vi "Autonomous Independent.vi"   [LabVIEW 2015]
doc: "This VI is called when autonomous begins, and will automatically be terminated when autonomous ends. You can carry out timed or sensor driven robot movement independently without needing to return to the caller."
uses:
  <vilib>/Rock Robotics/WPI/Solenoid/WPI_SolenoidValue.ctl
  <vilib>/Rock Robotics/WPI/Utilities/WPI_GetSetVariantRefNum.vi
  <vilib>/Rock Robotics/Network Tables/NT Read String.vi
  <vilib>/Rock Robotics/WPI/Solenoid/WPI_SolenoidSetEnum.vi
  Robot Global Data.vi
  <vilib>/Rock Robotics/Network Tables/NT Write Numeric Array.vi
panel:
  # "Be sure to right-click and choose Data Operations>>Make Current Value default if you want to save the array values with the VI"
types:
  T1 = typedef "WPI_JoystickDevRef.ctl" = cluster{"Device":T2}
  T2 = typedef "WPI_JoystickDeviceEnum.ctl" = enum16{"USB 0", "USB 1", "USB 2", "USB 3", "USB 4", "USB 5"}
  T3 = typedef "WPI_SolenoidValue.ctl" = enum16{"Off", "On", "Forward", "Reverse"}
  T4 = typedef "WPI_SolenoidDevRef.ctl" = cluster{"DevStatus":errorcluster, "Pneumatics Control Module":u8, "Forward Solenoid Channel":T5, "Reverse Solenoid Channel":T5}
  T5 = typedef "WPI_SolenoidChannel.ctl" = enum8{"Solenoid 0", "Solenoid 1", "Solenoid 2", "Solenoid 3", "Solenoid 4", "Solenoid 5", "Solenoid 6", "Solenoid 7", "Invalid"}
  T6 = typedef "WPI_RobotDriveDevRef.ctl" = cluster{"DevStatus":errorcluster, "Motors[]":T7[], "Square Inputs":bool, "Max Output":dbl}
  T7 = typedef "WPI_MotorControlDeviceRef.ctl" = cluster{"DeviceStatus":errorcluster, "Type":T8, "PWM":cluster{"PWM Channel":T9, "DeadBand":T10}, "CAN":cluster{"Device Number":u8, "Control Mode":T11, "Semaphore":T12, "Max Vout":dbl, "TalonSRX Control Mode":T13}, "Invert":bool}
  T8 = typedef "WPI_MotorControlType.ctl" = enum16{"PWM", "CAN", "CANTalonSRX"}
  T9 = typedef "FPGA_DIOPWMChannel.ctl" = enum8{"PWM 0", "PWM 1", "PWM 2", "PWM 3", "PWM 4", "PWM 5", "PWM 6", "PWM 7", "PWM 8", "PWM 9", "PWM MXP 0", "PWM MXP 1", "PWM MXP 2", "PWM MXP 3", "PWM MXP 4", "PWM MXP 5", "PWM MXP 6", "PWM MXP 7", "PWM MXP 8", "PWM MXP 9", "Invalid"}
  T10 = typedef "WPI_PWMDeadband.ctl" = cluster{"Name":string, "maxPositivePwm":i32, "minPositivePwm":i32, "centerPwm":i32, "maxNegativePwm":i32, "minNegativePwm":i32, "angularRange":u16}
  T11 = typedef "WPI_CANJaguar_ControlMode.ctl" = enum8{"Percent VBus", "Current", "Speed", "Position", "Voltage"}
  T12 = typedef "Semaphore RefNum" = refnum<k1>
  T13 = typedef "WPI_CANTalonSRX_APIControlMode.ctl" = enum8{"Percent VBus", "Speed", "Position", "Slave", "Unchanged / Invalid", "Voltage Compensation", "Current", "Motion Profile"}
  T14 = typedef "WPI_DigitalInputDevRef.ctl" = cluster{"DevStatus":errorcluster, "DIO Channel":T15}
  T15 = typedef "FPGA_DIOChannel.ctl" = enum8{"DIO 0", "DIO 1", "DIO 2", "DIO 3", "DIO 4", "DIO 5", "DIO 6", "DIO 7", "DIO 8", "DIO 9", "DIO MXP 0", "DIO MXP 1", "DIO MXP 2", "DIO MXP 3", "DIO MXP 4", "DIO MXP 5", "DIO MXP 6", "DIO MXP 7", "DIO MXP 8", "DIO MXP 9", "DIO MXP 10", "DIO MXP 11", "DIO MXP 12", "DIO MXP 13", "DIO MXP 14", "DIO MXP 15", "Invalid"}
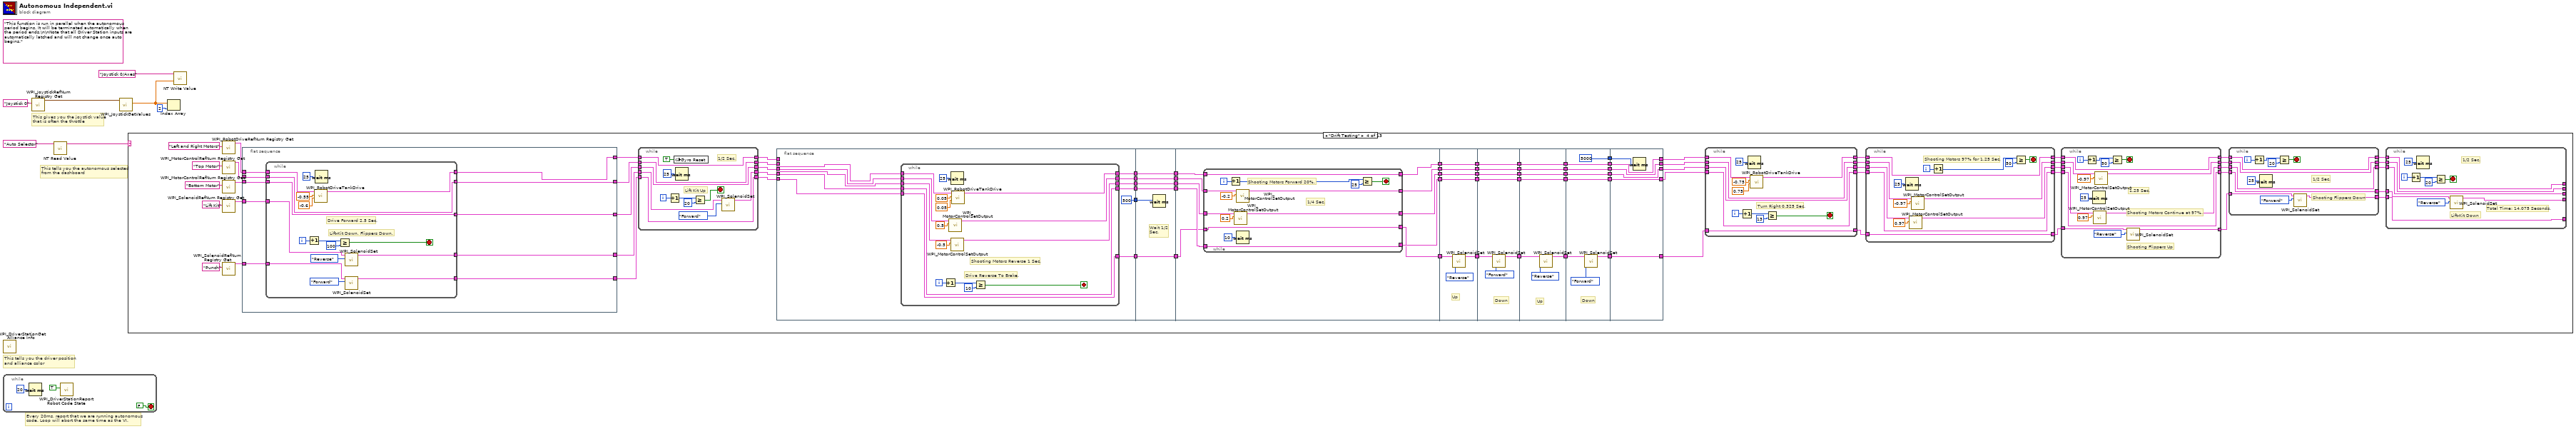
[diagram p0: block diagram]
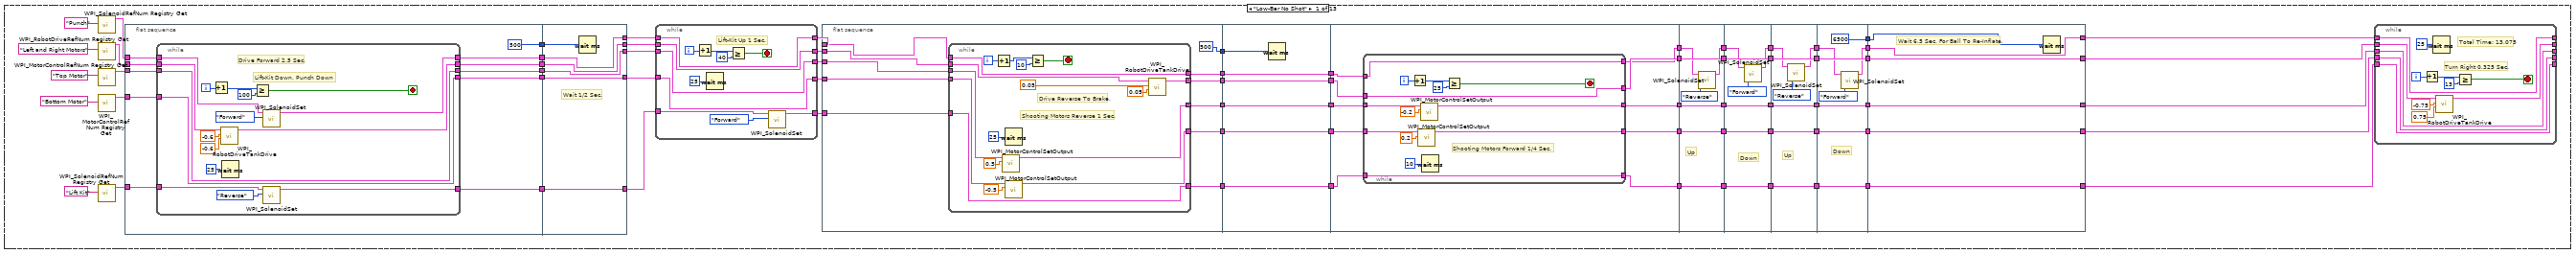
[diagram p2: hidden frame]
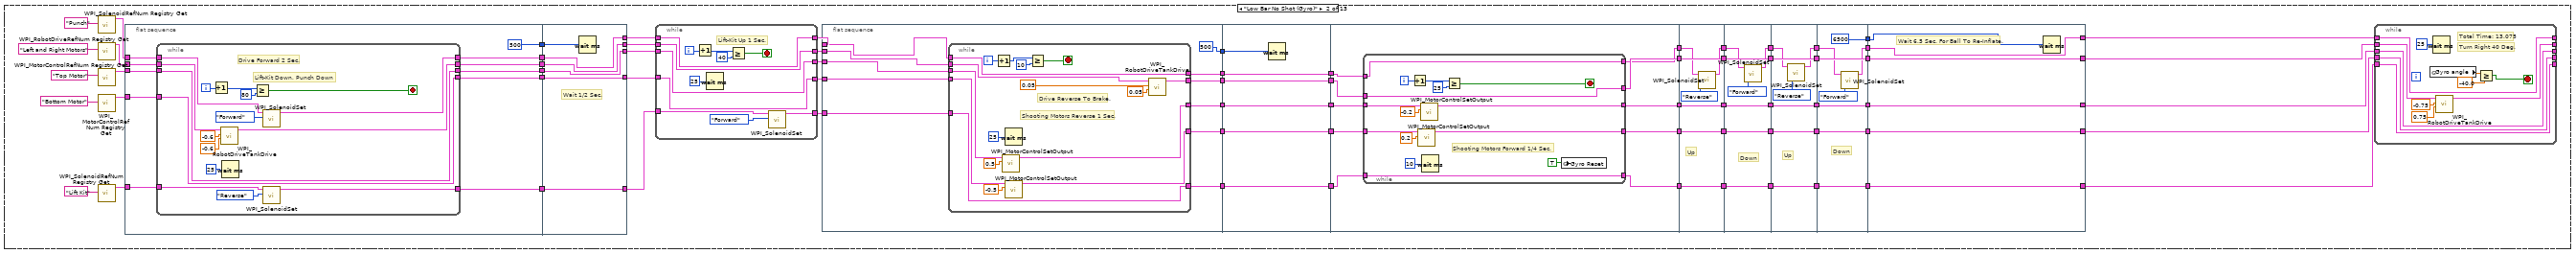
[diagram p3: hidden frame]
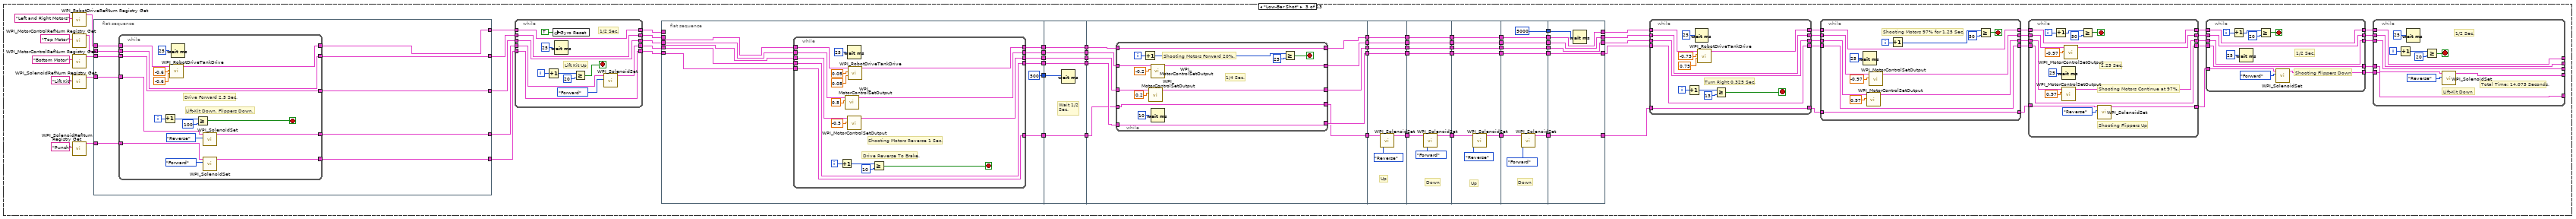
[diagram p4: hidden frame]
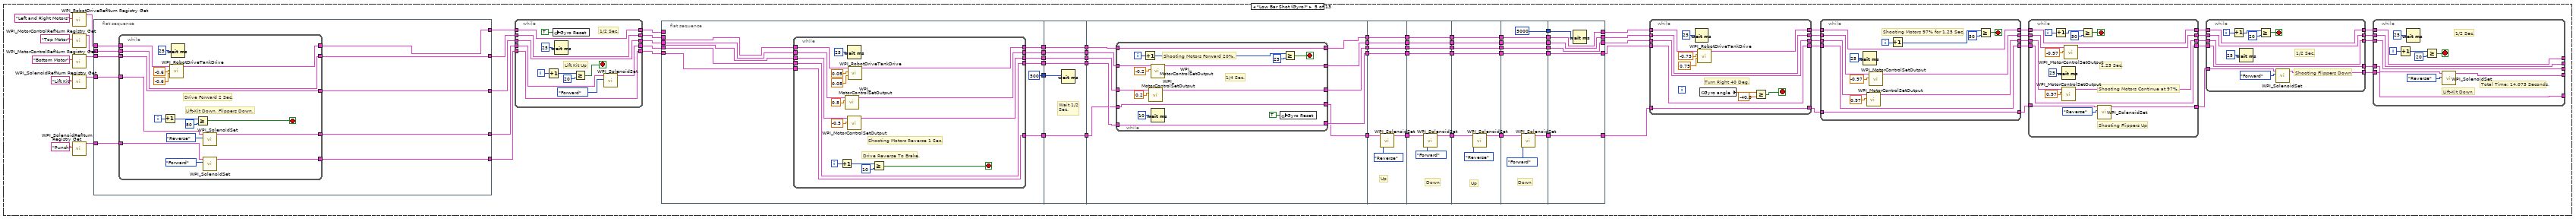
[diagram p5: hidden frame]
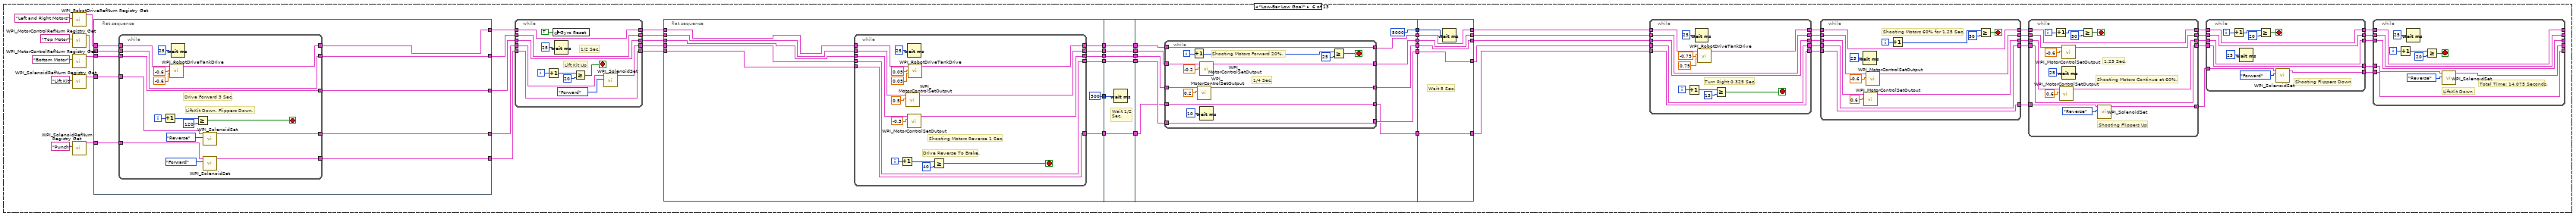
[diagram p6: hidden frame]
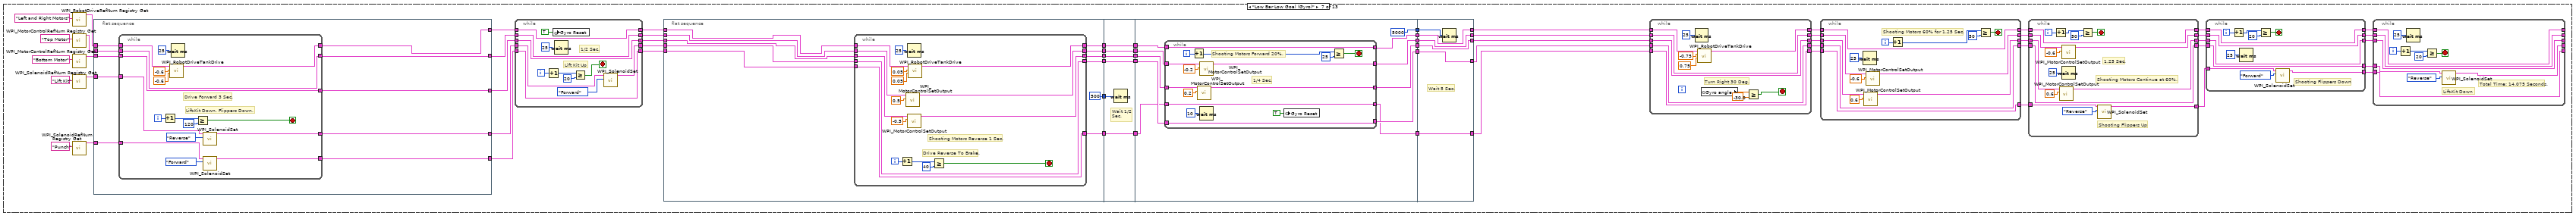
[diagram p7: hidden frame]
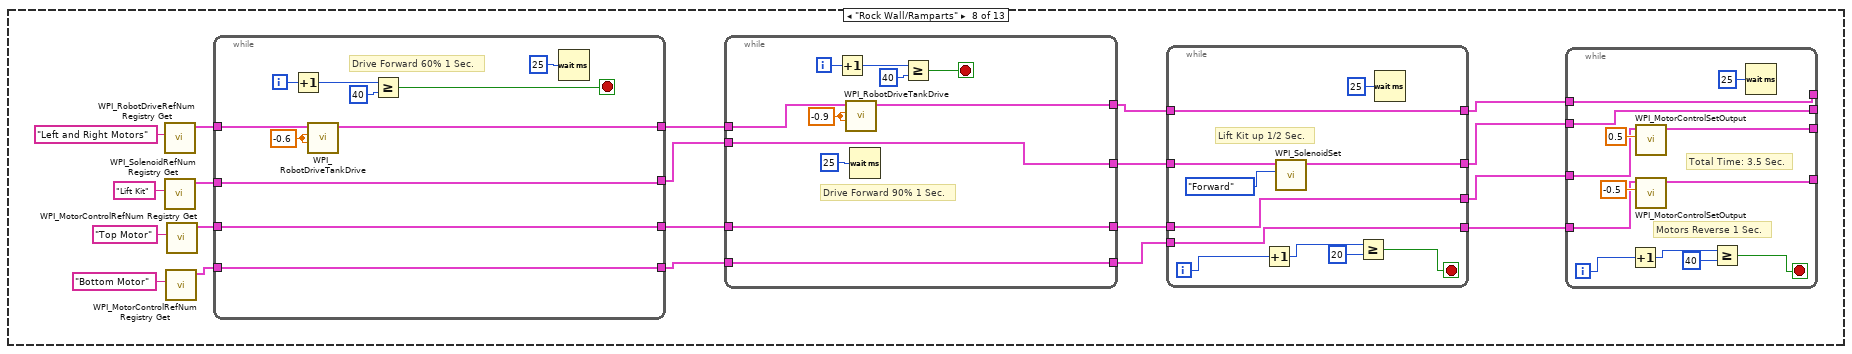
[diagram p8: hidden frame]
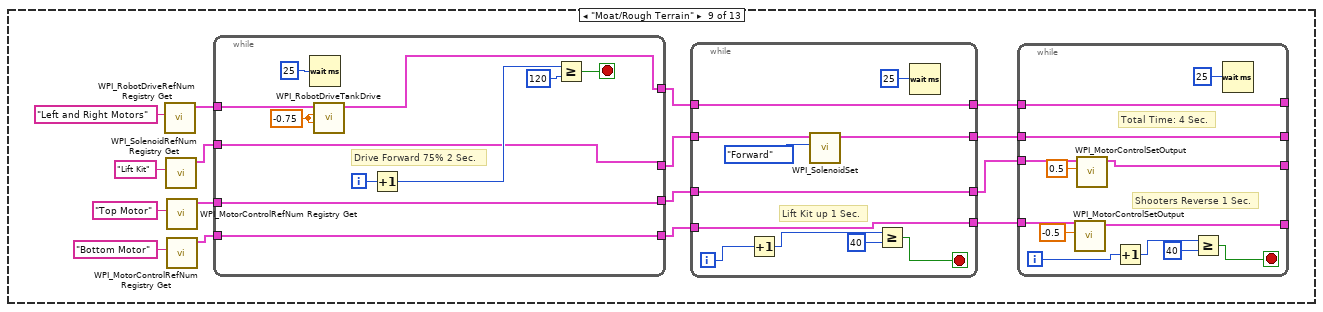
[diagram p9: hidden frame]
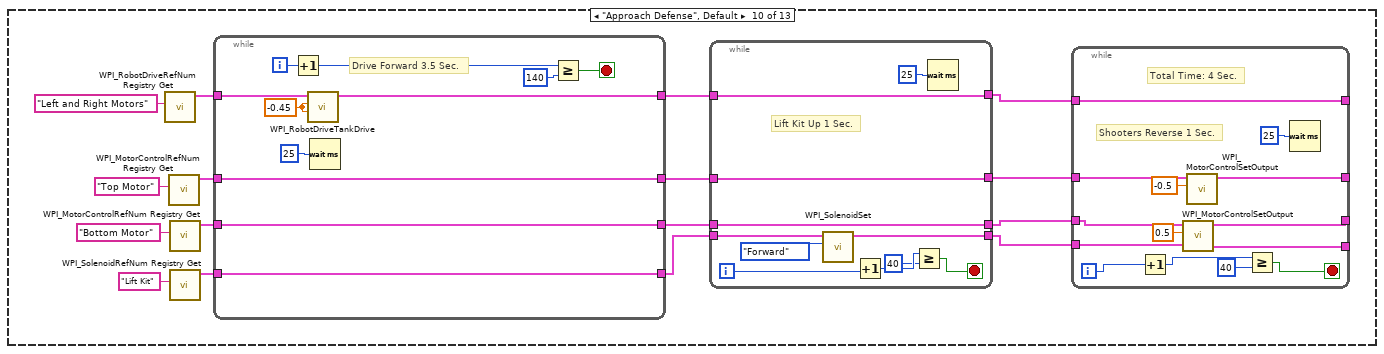
[diagram p10: hidden frame]
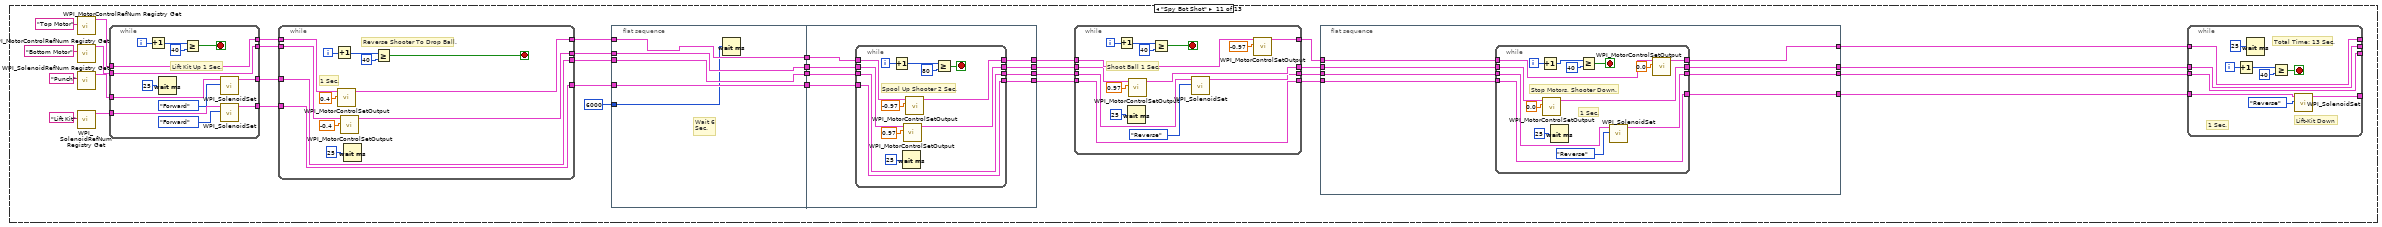
[diagram p11: hidden frame]
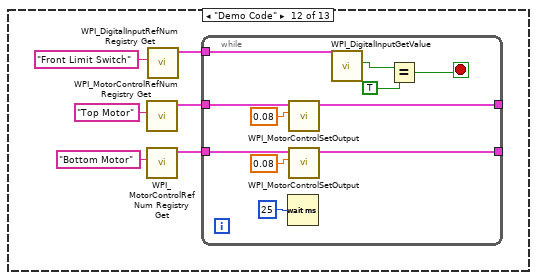
[diagram p12: hidden frame]
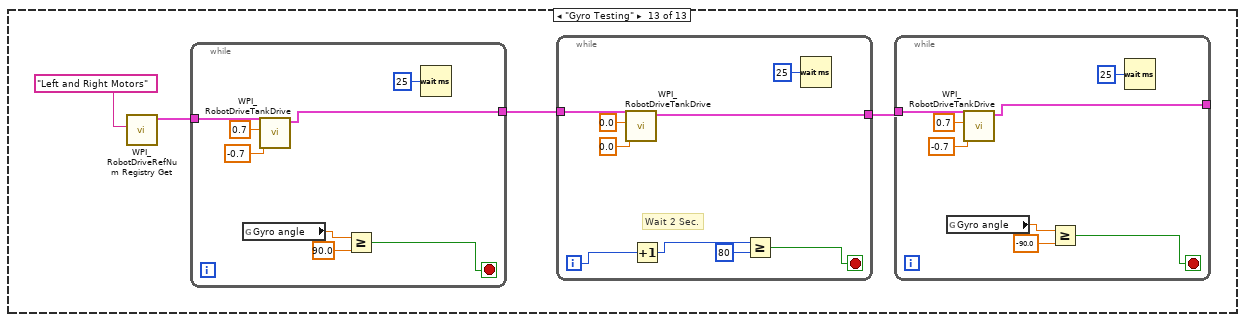
[diagram p13: hidden frame]
diagram:
  (unwired) "This function is run in parallel when the autonomous period begins. It will be terminated automatically when the period ends.\n\nNote that all Driver Station inputs are automatically latched and will not change once auto begins."
  # "This tells you the autonomous selected\nfrom the dashboard"
  # "Every 20ms, report that we are running autonomous\ncode. Loop will abort the same time as the VI."
  # "This gives you the joystick value\nthat is often the throttle"
  # "This tells you the driver position\nand alliance color"
  n1 = call <vilib>:"WPI_DriverStationGet Alliance Info.vi"() -> ()  [unwired: 12 out]
  n2 = while {
    stop <- FALSE stop-if-true
    n3 = Wait (ms)(milliseconds to wait=u32 20) -> ()  [unwired: 1 out]
    n4 = call <vilib>:"WPI_DriverStationReport Robot Code State.vi"("Autonomous"=TRUE) -> ()  [unwired: 10 in, 1 out]
  }
  n5 = call <vilib>:"WPI_JoystickRefNum Registry Get.vi"("refnum name"="Joystick 0") -> ("JoystickDevRef"=w6:T1)  [unwired: 1 in, 9 out]
  n6 = call-poly <vilib>:"NT Read Value.vi"("Name"="Auto Selector") -> ("String"=w3:string)  [unwired: 9 in, 1 out]
  n7 = call <vilib>:"WPI_JoystickGetValues.vi"("JoystickDevRef"=w6) -> ("Axes"=w2:dbl[])  [unwired: 6 in, 4 out]
  n8 = case shown="\"Drift Testing\"" w3 {
    frame "Low-Bar No Shot" {
      n9 = call <vilib>:"WPI_SolenoidRefNum Registry Get.vi"("refnum name"="Punch") -> ("SolenoidDevRef"=w70:T4)  [unwired: 9 in, 1 out]
      n10 = call <vilib>:"WPI_RobotDriveRefNum Registry Get.vi"("refnum name"="Left and Right Motors") -> ("RobotDriveDevRef"=w78:T6)  [unwired: 9 in, 1 out]
      n11 = call <vilib>:"WPI_MotorControlRefNum Registry Get.vi"("refnum name"="Top Motor") -> ("MotorControlDevRef"=w76:T7)  [unwired: 9 in, 1 out]
      n12 = call <vilib>:"WPI_MotorControlRefNum Registry Get.vi"("refnum name"="Bottom Motor") -> ("MotorControlDevRef"=w74:T7)  [unwired: 9 in, 1 out]
      n13 = call <vilib>:"WPI_SolenoidRefNum Registry Get.vi"("refnum name"="Lift Kit") -> ("SolenoidDevRef"=w72:T4)  [unwired: 9 in, 1 out]
      n14 = flat-sequence {
        tunnel: w78 -> [w89]
        tunnel: w76 -> [w87]
        tunnel: w74 -> [w85]
        tunnel: w72 -> [w83]
        tunnel: w70 -> [w81]
        tunnel: [w88] -> w53
        tunnel: [w86] -> w52
        tunnel: [w84] -> w51
        tunnel: [w82] -> w50
        tunnel: [w80] -> w49
        tunnel: [u32 500 ("milliseconds to wait")] -> w48
        tunnel: [w108] -> w69
        tunnel: [w109] -> w71
        tunnel: [w110] -> w73
        tunnel: [w111] -> w75
        tunnel: [w112] -> w77
        tunnel: w53 -> [w112]
        tunnel: w52 -> [w111]
        tunnel: w51 -> [w110]
        tunnel: w50 -> [w109]
        tunnel: w49 -> [w108]
        tunnel: w48 -> [w107]
        frame #0 {
          n15 = while {
            tunnel: w89 -> [w106]
            tunnel: [w99] -> w88
            tunnel: w87 -> [w97]
            tunnel: [w97] -> w86
            tunnel: w85 -> [w96]
            tunnel: [w96] -> w84
            tunnel: w83 -> [w95]
            tunnel: [w94] -> w82
            tunnel: [w90] -> w80
            tunnel: w81 -> [w91]
            i -> [w100]
            stop <- w101 stop-if-true
            # "Lift-Kit Down, Punch Down"
            # "Drive Forward 2.5 Sec."
            n16 = Increment(x=w100) -> (x+1=w103:i32)
            n17 = call <vilib>:"WPI_RobotDriveTankDrive.vi"("Right axis value"=-0.6, "Left axis value"=-0.6, "RobotDriveDevRef"=w106) -> ("RobotDriveDevRef"=w99:T6)  [unwired: 6 in, 2 out]
            n18 = Wait (ms)(milliseconds to wait=u32 25) -> ()  [unwired: 1 out]
            n19 = Greater Or Equal?(x=w103, y=100) -> (x >= y?=w101:bool)
            n20 = call-poly <vilib>:"WPI_SolenoidSet.vi"("Value"=WPI_SolenoidValue."Forward", "SolenoidDevRef"=w91) -> ("SolenoidDevRef"=w90:T4)  [unwired: 8 in, 1 out]
            n21 = call-poly <vilib>:"WPI_SolenoidSet.vi"("Value"=WPI_SolenoidValue."Reverse", "SolenoidDevRef"=w95) -> ("SolenoidDevRef"=w94:T4)  [unwired: 8 in, 1 out]
          }
        }
        frame #1 {
          # "Wait 1/2 Sec."
          n22 = Wait (ms)(milliseconds to wait=w107) -> ()  [unwired: 1 out]
        }
      }
      n23 = while {
        tunnel: [w217] -> w68
        tunnel: w77 -> [w217]
        tunnel: [w211] -> w64
        tunnel: w75 -> [w211]
        tunnel: [w210] -> w63
        tunnel: w73 -> [w210]
        tunnel: w71 -> [w208]
        tunnel: [w207] -> w62
        tunnel: w69 -> [w206]
        tunnel: [w206] -> w66
        i -> [w213]
        stop <- w214 stop-if-true
        # "Lift-Kit Up 1 Sec."
        n24 = Increment(x=w213) -> (x+1=w215:i32)
        n25 = Wait (ms)(milliseconds to wait=u32 25) -> ()  [unwired: 1 out]
        n26 = Greater Or Equal?(x=w215, y=40) -> (x >= y?=w214:bool)
        n27 = call-poly <vilib>:"WPI_SolenoidSet.vi"("Value"=WPI_SolenoidValue."Forward", "SolenoidDevRef"=w208) -> ("SolenoidDevRef"=w207:T4)  [unwired: 8 in, 1 out]
      }
      n28 = flat-sequence {
        tunnel: [w122] -> w47
        tunnel: [w121] -> w45
        tunnel: [w117] -> w43
        tunnel: [w116] -> w41
        tunnel: [w115] -> w39
        tunnel: [u32 500 ("milliseconds to wait")] -> w37
        tunnel: w62 -> [w118]
        tunnel: w63 -> [w119]
        tunnel: w64 -> [w120]
        tunnel: w66 -> [w114]
        tunnel: w68 -> [w123]
        tunnel: w47 -> [w146]
        tunnel: [w146] -> w46
        tunnel: w45 -> [w145]
        tunnel: [w145] -> w44
        tunnel: w43 -> [w144]
        tunnel: [w144] -> w42
        tunnel: w41 -> [w143]
        tunnel: [w143] -> w40
        tunnel: w39 -> [w142]
        tunnel: [w142] -> w38
        tunnel: w37 -> [w141]
        tunnel: w46 -> [w152]
        tunnel: [w151] -> w36
        tunnel: w44 -> [w150]
        tunnel: [w149] -> w35
        tunnel: w42 -> [w148]
        tunnel: [w147] -> w34
        tunnel: w40 -> [w156]
        tunnel: [w154] -> w33
        tunnel: w38 -> [w155]
        tunnel: [w153] -> w32
        tunnel: w36 -> [w177]
        tunnel: [w177] -> w31
        tunnel: w35 -> [w176]
        tunnel: [w172] -> w30
        tunnel: w34 -> [w175]
        tunnel: [w175] -> w29
        tunnel: w33 -> [w174]
        tunnel: [w174] -> w28
        tunnel: w32 -> [w173]
        tunnel: [w173] -> w27
        tunnel: w31 -> [w184]
        tunnel: [w184] -> w26
        tunnel: w30 -> [w183]
        tunnel: [w179] -> w25
        tunnel: w29 -> [w182]
        tunnel: [w182] -> w24
        tunnel: w28 -> [w181]
        tunnel: [w181] -> w23
        tunnel: w27 -> [w180]
        tunnel: [w180] -> w22
        tunnel: w26 -> [w191]
        tunnel: [w191] -> w21
        tunnel: w25 -> [w190]
        tunnel: [w186] -> w19
        tunnel: w24 -> [w189]
        tunnel: [w189] -> w17
        tunnel: w23 -> [w188]
        tunnel: [w188] -> w15
        tunnel: w22 -> [w187]
        tunnel: [w187] -> w13
        tunnel: w21 -> [w199]
        tunnel: [w199] -> w20
        tunnel: w19 -> [w198]
        tunnel: [w194] -> w18
        tunnel: w17 -> [w197]
        tunnel: [w197] -> w16
        tunnel: w15 -> [w196]
        tunnel: [w196] -> w14
        tunnel: w13 -> [w195]
        tunnel: [w195] -> w12
        tunnel: [u32 6500 ("milliseconds to wait")] -> w11
        tunnel: [w201] -> w59
        tunnel: [w202] -> w60
        tunnel: [w203] -> w61
        tunnel: [w204] -> w65
        tunnel: [w205] -> w67
        tunnel: w20 -> [w205]
        tunnel: w18 -> [w204]
        tunnel: w16 -> [w203]
        tunnel: w14 -> [w202]
        tunnel: w12 -> [w201]
        tunnel: w11 -> [w200]
        frame #0 {
          n29 = while {
            tunnel: [w127] -> w122
            tunnel: w123 -> [w140]
            tunnel: [w124] -> w121
            tunnel: w114 -> [w124]
            tunnel: w120 -> [w139]
            tunnel: w119 -> [w138]
            tunnel: [w135] -> w117
            tunnel: w118 -> [w135]
            tunnel: [w134] -> w116
            tunnel: [w133] -> w115
            i -> [w129]
            stop <- w128 stop-if-true
            # "Drive Reverse To Brake."
            # "Shooting Motors Reverse 1 Sec."
            n30 = Increment(x=w129) -> (x+1=w131:i32)
            n31 = call <vilib>:"WPI_MotorControlSetOutput.vi"("Output"=0.5, "MotorControlDevRef"=w139) -> ("MotorControlDevRef"=w134:T7)  [unwired: 7 in, 2 out]
            n32 = Wait (ms)(milliseconds to wait=u32 25) -> ()  [unwired: 1 out]
            n33 = call <vilib>:"WPI_MotorControlSetOutput.vi"("Output"=-0.5, "MotorControlDevRef"=w138) -> ("MotorControlDevRef"=w133:T7)  [unwired: 7 in, 2 out]
            n34 = Greater Or Equal?(x=w131, y=10) -> (x >= y?=w128:bool)
            n35 = call <vilib>:"WPI_RobotDriveTankDrive.vi"("Right axis value"=0.05, "Left axis value"=0.05, "RobotDriveDevRef"=w140) -> ("RobotDriveDevRef"=w127:T6)  [unwired: 6 in, 2 out]
          }
        }
        frame #1 {
          n36 = Wait (ms)(milliseconds to wait=w141) -> ()  [unwired: 1 out]
        }
        frame #2 {
          n37 = while {
            tunnel: w156 -> [w170]
            tunnel: w155 -> [w169]
            tunnel: [w161] -> w154
            tunnel: [w160] -> w153
            tunnel: [w159] -> w151
            tunnel: w152 -> [w159]
            tunnel: [w158] -> w149
            tunnel: w150 -> [w158]
            tunnel: [w157] -> w147
            tunnel: w148 -> [w157]
            i -> [w165]
            stop <- w162 stop-if-true
            # "Shooting Motors Forward 1/4 Sec."
            n38 = Increment(x=w165) -> (x+1=w164:i32)
            n39 = call <vilib>:"WPI_MotorControlSetOutput.vi"("Output"=0.2, "MotorControlDevRef"=w169) -> ("MotorControlDevRef"=w160:T7)  [unwired: 7 in, 2 out]
            n40 = call <vilib>:"WPI_MotorControlSetOutput.vi"("Output"=-0.2, "MotorControlDevRef"=w170) -> ("MotorControlDevRef"=w161:T7)  [unwired: 7 in, 2 out]
            n41 = Wait (ms)(milliseconds to wait=u32 10) -> ()  [unwired: 1 out]
            n42 = Greater Or Equal?(x=w164, y=25) -> (x >= y?=w162:bool)
          }
        }
        frame #3 {
          # "Up"
          n43 = call-poly <vilib>:"WPI_SolenoidSet.vi"("Value"=WPI_SolenoidValue."Reverse", "SolenoidDevRef"=w176) -> ("SolenoidDevRef"=w172:T4)  [unwired: 8 in, 1 out]
        }
        frame #4 {
          # "Down"
          n44 = call-poly <vilib>:"WPI_SolenoidSet.vi"("Value"=WPI_SolenoidValue."Forward", "SolenoidDevRef"=w183) -> ("SolenoidDevRef"=w179:T4)  [unwired: 8 in, 1 out]
        }
        frame #5 {
          # "Up"
          n45 = call-poly <vilib>:"WPI_SolenoidSet.vi"("Value"=WPI_SolenoidValue."Reverse", "SolenoidDevRef"=w190) -> ("SolenoidDevRef"=w186:T4)  [unwired: 8 in, 1 out]
        }
        frame #6 {
          # "Down"
          n46 = call-poly <vilib>:"WPI_SolenoidSet.vi"("Value"=WPI_SolenoidValue."Forward", "SolenoidDevRef"=w198) -> ("SolenoidDevRef"=w194:T4)  [unwired: 8 in, 1 out]
        }
        frame #7 {
          # "Wait 6.5 Sec. For Ball To Re-Inflate."
          n47 = Wait (ms)(milliseconds to wait=w200) -> ()  [unwired: 1 out]
        }
      }
      n48 = while {
        tunnel: w67 -> [w230]
        tunnel: w60 -> [w226]
        tunnel: [w226] -> _
        tunnel: [w225] -> _
        tunnel: w59 -> [w225]
        tunnel: [w224] -> _
        tunnel: [w223] -> _
        tunnel: w61 -> [w223]
        tunnel: [w222] -> _
        tunnel: w65 -> [w222]
        i -> [w220]
        stop <- w218 stop-if-true
        # "Total Time: 13.075"
        # "Turn Right 0.325 Sec."
        n49 = Increment(x=w220) -> (x+1=w221:i32)
        n50 = Wait (ms)(milliseconds to wait=u32 25) -> ()  [unwired: 1 out]
        n51 = call <vilib>:"WPI_RobotDriveTankDrive.vi"("Right axis value"=0.75, "Left axis value"=-0.75, "RobotDriveDevRef"=w230) -> ("RobotDriveDevRef"=w224:T6)  [unwired: 6 in, 2 out]
        n52 = Greater Or Equal?(x=w221, y=13) -> (x >= y?=w218:bool)
      }
    }
    frame "Low Bar No Shot (Gyro)" {
      n53 = call <vilib>:"WPI_SolenoidRefNum Registry Get.vi"("refnum name"="Punch") -> ("SolenoidDevRef"=w290:T4)  [unwired: 9 in, 1 out]
      n54 = call <vilib>:"WPI_RobotDriveRefNum Registry Get.vi"("refnum name"="Left and Right Motors") -> ("RobotDriveDevRef"=w298:T6)  [unwired: 9 in, 1 out]
      n55 = call <vilib>:"WPI_MotorControlRefNum Registry Get.vi"("refnum name"="Top Motor") -> ("MotorControlDevRef"=w296:T7)  [unwired: 9 in, 1 out]
      n56 = call <vilib>:"WPI_MotorControlRefNum Registry Get.vi"("refnum name"="Bottom Motor") -> ("MotorControlDevRef"=w294:T7)  [unwired: 9 in, 1 out]
      n57 = call <vilib>:"WPI_SolenoidRefNum Registry Get.vi"("refnum name"="Lift Kit") -> ("SolenoidDevRef"=w292:T4)  [unwired: 9 in, 1 out]
      n58 = flat-sequence {
        tunnel: w298 -> [w309]
        tunnel: w296 -> [w307]
        tunnel: w294 -> [w305]
        tunnel: w292 -> [w303]
        tunnel: w290 -> [w301]
        tunnel: [w308] -> w273
        tunnel: [w306] -> w272
        tunnel: [w304] -> w271
        tunnel: [w302] -> w270
        tunnel: [w300] -> w269
        tunnel: [u32 500 ("milliseconds to wait")] -> w268
        tunnel: [w328] -> w289
        tunnel: [w329] -> w291
        tunnel: [w330] -> w293
        tunnel: [w331] -> w295
        tunnel: [w332] -> w297
        tunnel: w273 -> [w332]
        tunnel: w272 -> [w331]
        tunnel: w271 -> [w330]
        tunnel: w270 -> [w329]
        tunnel: w269 -> [w328]
        tunnel: w268 -> [w327]
        frame #0 {
          n59 = while {
            tunnel: w309 -> [w326]
            tunnel: [w319] -> w308
            tunnel: w307 -> [w317]
            tunnel: [w317] -> w306
            tunnel: w305 -> [w316]
            tunnel: [w316] -> w304
            tunnel: w303 -> [w315]
            tunnel: [w314] -> w302
            tunnel: [w310] -> w300
            tunnel: w301 -> [w311]
            i -> [w320]
            stop <- w321 stop-if-true
            # "Lift-Kit Down, Punch Down"
            # "Drive Forward 2 Sec."
            n60 = Increment(x=w320) -> (x+1=w323:i32)
            n61 = call <vilib>:"WPI_RobotDriveTankDrive.vi"("Right axis value"=-0.6, "Left axis value"=-0.6, "RobotDriveDevRef"=w326) -> ("RobotDriveDevRef"=w319:T6)  [unwired: 6 in, 2 out]
            n62 = Wait (ms)(milliseconds to wait=u32 25) -> ()  [unwired: 1 out]
            n63 = Greater Or Equal?(x=w323, y=80) -> (x >= y?=w321:bool)
            n64 = call-poly <vilib>:"WPI_SolenoidSet.vi"("Value"=WPI_SolenoidValue."Forward", "SolenoidDevRef"=w311) -> ("SolenoidDevRef"=w310:T4)  [unwired: 8 in, 1 out]
            n65 = call-poly <vilib>:"WPI_SolenoidSet.vi"("Value"=WPI_SolenoidValue."Reverse", "SolenoidDevRef"=w315) -> ("SolenoidDevRef"=w314:T4)  [unwired: 8 in, 1 out]
          }
        }
        frame #1 {
          # "Wait 1/2 Sec."
          n66 = Wait (ms)(milliseconds to wait=w327) -> ()  [unwired: 1 out]
        }
      }
      n67 = while {
        tunnel: [w438] -> w288
        tunnel: w297 -> [w438]
        tunnel: [w432] -> w284
        tunnel: w295 -> [w432]
        tunnel: [w431] -> w283
        tunnel: w293 -> [w431]
        tunnel: w291 -> [w429]
        tunnel: [w428] -> w282
        tunnel: w289 -> [w427]
        tunnel: [w427] -> w286
        i -> [w434]
        stop <- w435 stop-if-true
        # "Lift-Kit Up 1 Sec."
        n68 = Increment(x=w434) -> (x+1=w436:i32)
        n69 = Wait (ms)(milliseconds to wait=u32 25) -> ()  [unwired: 1 out]
        n70 = Greater Or Equal?(x=w436, y=40) -> (x >= y?=w435:bool)
        n71 = call-poly <vilib>:"WPI_SolenoidSet.vi"("Value"=WPI_SolenoidValue."Forward", "SolenoidDevRef"=w429) -> ("SolenoidDevRef"=w428:T4)  [unwired: 8 in, 1 out]
      }
      n72 = flat-sequence {
        tunnel: [w342] -> w267
        tunnel: [w341] -> w265
        tunnel: [w337] -> w263
        tunnel: [w336] -> w261
        tunnel: [w335] -> w259
        tunnel: [u32 500 ("milliseconds to wait")] -> w257
        tunnel: w282 -> [w338]
        tunnel: w283 -> [w339]
        tunnel: w284 -> [w340]
        tunnel: w286 -> [w334]
        tunnel: w288 -> [w343]
        tunnel: w267 -> [w366]
        tunnel: [w366] -> w266
        tunnel: w265 -> [w365]
        tunnel: [w365] -> w264
        tunnel: w263 -> [w364]
        tunnel: [w364] -> w262
        tunnel: w261 -> [w363]
        tunnel: [w363] -> w260
        tunnel: w259 -> [w362]
        tunnel: [w362] -> w258
        tunnel: w257 -> [w361]
        tunnel: w266 -> [w372]
        tunnel: [w371] -> w256
        tunnel: w264 -> [w370]
        tunnel: [w369] -> w255
        tunnel: w262 -> [w368]
        tunnel: [w367] -> w254
        tunnel: w260 -> [w376]
        tunnel: [w374] -> w253
        tunnel: w258 -> [w375]
        tunnel: [w373] -> w252
        tunnel: w256 -> [w398]
        tunnel: [w398] -> w251
        tunnel: w255 -> [w397]
        tunnel: [w393] -> w250
        tunnel: w254 -> [w396]
        tunnel: [w396] -> w249
        tunnel: w253 -> [w395]
        tunnel: [w395] -> w248
        tunnel: w252 -> [w394]
        tunnel: [w394] -> w247
        tunnel: w251 -> [w405]
        tunnel: [w405] -> w246
        tunnel: w250 -> [w404]
        tunnel: [w400] -> w245
        tunnel: w249 -> [w403]
        tunnel: [w403] -> w244
        tunnel: w248 -> [w402]
        tunnel: [w402] -> w243
        tunnel: w247 -> [w401]
        tunnel: [w401] -> w242
        tunnel: w246 -> [w412]
        tunnel: [w412] -> w241
        tunnel: w245 -> [w411]
        tunnel: [w407] -> w239
        tunnel: w244 -> [w410]
        tunnel: [w410] -> w237
        tunnel: w243 -> [w409]
        tunnel: [w409] -> w235
        tunnel: w242 -> [w408]
        tunnel: [w408] -> w233
        tunnel: w241 -> [w420]
        tunnel: [w420] -> w240
        tunnel: w239 -> [w419]
        tunnel: [w415] -> w238
        tunnel: w237 -> [w418]
        tunnel: [w418] -> w236
        tunnel: w235 -> [w417]
        tunnel: [w417] -> w234
        tunnel: w233 -> [w416]
        tunnel: [w416] -> w232
        tunnel: [u32 6500 ("milliseconds to wait")] -> w231
        tunnel: [w422] -> w279
        tunnel: [w423] -> w280
        tunnel: [w424] -> w281
        tunnel: [w425] -> w285
        tunnel: [w426] -> w287
        tunnel: w240 -> [w426]
        tunnel: w238 -> [w425]
        tunnel: w236 -> [w424]
        tunnel: w234 -> [w423]
        tunnel: w232 -> [w422]
        tunnel: w231 -> [w421]
        frame #0 {
          n73 = while {
            tunnel: [w347] -> w342
            tunnel: w343 -> [w360]
            tunnel: [w344] -> w341
            tunnel: w334 -> [w344]
            tunnel: w340 -> [w359]
            tunnel: w339 -> [w358]
            tunnel: [w355] -> w337
            tunnel: w338 -> [w355]
            tunnel: [w354] -> w336
            tunnel: [w353] -> w335
            i -> [w349]
            stop <- w348 stop-if-true
            # "Drive Reverse To Brake."
            # "Shooting Motors Reverse 1 Sec."
            n74 = Increment(x=w349) -> (x+1=w351:i32)
            n75 = call <vilib>:"WPI_MotorControlSetOutput.vi"("Output"=0.5, "MotorControlDevRef"=w359) -> ("MotorControlDevRef"=w354:T7)  [unwired: 7 in, 2 out]
            n76 = Wait (ms)(milliseconds to wait=u32 25) -> ()  [unwired: 1 out]
            n77 = call <vilib>:"WPI_MotorControlSetOutput.vi"("Output"=-0.5, "MotorControlDevRef"=w358) -> ("MotorControlDevRef"=w353:T7)  [unwired: 7 in, 2 out]
            n78 = Greater Or Equal?(x=w351, y=10) -> (x >= y?=w348:bool)
            n79 = call <vilib>:"WPI_RobotDriveTankDrive.vi"("Right axis value"=0.05, "Left axis value"=0.05, "RobotDriveDevRef"=w360) -> ("RobotDriveDevRef"=w347:T6)  [unwired: 6 in, 2 out]
          }
        }
        frame #1 {
          n80 = Wait (ms)(milliseconds to wait=w361) -> ()  [unwired: 1 out]
        }
        frame #2 {
          n81 = while {
            tunnel: w376 -> [w391]
            tunnel: w375 -> [w390]
            tunnel: [w382] -> w374
            tunnel: [w381] -> w373
            tunnel: [w380] -> w371
            tunnel: w372 -> [w380]
            tunnel: [w379] -> w369
            tunnel: w370 -> [w379]
            tunnel: [w378] -> w367
            tunnel: w368 -> [w378]
            i -> [w386]
            stop <- w383 stop-if-true
            # "Shooting Motors Forward 1/4 Sec."
            n82 = Increment(x=w386) -> (x+1=w385:i32)
            n83 = call <vilib>:"WPI_MotorControlSetOutput.vi"("Output"=0.2, "MotorControlDevRef"=w390) -> ("MotorControlDevRef"=w381:T7)  [unwired: 7 in, 2 out]
            n84 = call <vilib>:"WPI_MotorControlSetOutput.vi"("Output"=-0.2, "MotorControlDevRef"=w391) -> ("MotorControlDevRef"=w382:T7)  [unwired: 7 in, 2 out]
            n85 = Wait (ms)(milliseconds to wait=u32 10) -> ()  [unwired: 1 out]
            n86 = Greater Or Equal?(x=w385, y=25) -> (x >= y?=w383:bool)
            n87 = global write "Robot Global Data.vi" "Gyro Reset"(TRUE ("Gyro Reset")) -> ()
          }
        }
        frame #3 {
          # "Up"
          n88 = call-poly <vilib>:"WPI_SolenoidSet.vi"("Value"=WPI_SolenoidValue."Reverse", "SolenoidDevRef"=w397) -> ("SolenoidDevRef"=w393:T4)  [unwired: 8 in, 1 out]
        }
        frame #4 {
          # "Down"
          n89 = call-poly <vilib>:"WPI_SolenoidSet.vi"("Value"=WPI_SolenoidValue."Forward", "SolenoidDevRef"=w404) -> ("SolenoidDevRef"=w400:T4)  [unwired: 8 in, 1 out]
        }
        frame #5 {
          # "Up"
          n90 = call-poly <vilib>:"WPI_SolenoidSet.vi"("Value"=WPI_SolenoidValue."Reverse", "SolenoidDevRef"=w411) -> ("SolenoidDevRef"=w407:T4)  [unwired: 8 in, 1 out]
        }
        frame #6 {
          # "Down"
          n91 = call-poly <vilib>:"WPI_SolenoidSet.vi"("Value"=WPI_SolenoidValue."Forward", "SolenoidDevRef"=w419) -> ("SolenoidDevRef"=w415:T4)  [unwired: 8 in, 1 out]
        }
        frame #7 {
          # "Wait 6.5 Sec. For Ball To Re-Inflate."
          n92 = Wait (ms)(milliseconds to wait=w421) -> ()  [unwired: 1 out]
        }
      }
      n93 = while {
        tunnel: w287 -> [w450]
        tunnel: w280 -> [w446]
        tunnel: [w446] -> _
        tunnel: [w445] -> _
        tunnel: w279 -> [w445]
        tunnel: [w444] -> _
        tunnel: [w443] -> _
        tunnel: w281 -> [w443]
        tunnel: [w442] -> _
        tunnel: w285 -> [w442]
        stop <- w440 stop-if-true
        # "Total Time: 13.075"
        # "Turn Right 40 Deg."
        n94 = global read "Robot Global Data.vi" "Gyro angle"() -> (w441:dbl)
        n95 = Wait (ms)(milliseconds to wait=u32 25) -> ()  [unwired: 1 out]
        n96 = call <vilib>:"WPI_RobotDriveTankDrive.vi"("Right axis value"=0.75, "Left axis value"=-0.75, "RobotDriveDevRef"=w450) -> ("RobotDriveDevRef"=w444:T6)  [unwired: 6 in, 2 out]
        n97 = Greater Or Equal?(x=w441, y=-40.0) -> (x >= y?=w440:bool)
      }
    }
    frame "Low-Bar Shot" {
      n98 = call <vilib>:"WPI_RobotDriveRefNum Registry Get.vi"("refnum name"="Left and Right Motors") -> ("RobotDriveDevRef"=w532:T6)  [unwired: 9 in, 1 out]
      n99 = call <vilib>:"WPI_MotorControlRefNum Registry Get.vi"("refnum name"="Top Motor") -> ("MotorControlDevRef"=w528:T7)  [unwired: 9 in, 1 out]
      n100 = call <vilib>:"WPI_MotorControlRefNum Registry Get.vi"("refnum name"="Bottom Motor") -> ("MotorControlDevRef"=w526:T7)  [unwired: 9 in, 1 out]
      n101 = call <vilib>:"WPI_SolenoidRefNum Registry Get.vi"("refnum name"="Lift Kit") -> ("SolenoidDevRef"=w523:T4)  [unwired: 9 in, 1 out]
      n102 = call <vilib>:"WPI_SolenoidRefNum Registry Get.vi"("refnum name"="Punch") -> ("SolenoidDevRef"=w520:T4)  [unwired: 9 in, 1 out]
      n103 = flat-sequence {
        tunnel: [w550] -> w519
        tunnel: [w551] -> w522
        tunnel: [w552] -> w525
        tunnel: [w553] -> w527
        tunnel: [w554] -> w529
        tunnel: w520 -> [w545]
        tunnel: w523 -> [w546]
        tunnel: w526 -> [w547]
        tunnel: w528 -> [w548]
        tunnel: w532 -> [w549]
        frame #0 {
          n104 = while {
            tunnel: w549 -> [w571]
            tunnel: [w564] -> w554
            tunnel: w548 -> [w562]
            tunnel: [w562] -> w553
            tunnel: w547 -> [w561]
            tunnel: [w561] -> w552
            tunnel: w546 -> [w560]
            tunnel: [w559] -> w551
            tunnel: [w555] -> w550
            tunnel: w545 -> [w556]
            i -> [w565]
            stop <- w566 stop-if-true
            # "Lift-Kit Down, Flippers Down."
            # "Drive Forward 2.5 Sec."
            n105 = Increment(x=w565) -> (x+1=w568:i32)
            n106 = call <vilib>:"WPI_RobotDriveTankDrive.vi"("Right axis value"=-0.6, "Left axis value"=-0.6, "RobotDriveDevRef"=w571) -> ("RobotDriveDevRef"=w564:T6)  [unwired: 6 in, 2 out]
            n107 = Wait (ms)(milliseconds to wait=u32 25) -> ()  [unwired: 1 out]
            n108 = Greater Or Equal?(x=w568, y=100) -> (x >= y?=w566:bool)
            n109 = call-poly <vilib>:"WPI_SolenoidSet.vi"("Value"=WPI_SolenoidValue."Reverse", "SolenoidDevRef"=w560) -> ("SolenoidDevRef"=w559:T4)  [unwired: 8 in, 1 out]
            n110 = call-poly <vilib>:"WPI_SolenoidSet.vi"("Value"=WPI_SolenoidValue."Forward", "SolenoidDevRef"=w556) -> ("SolenoidDevRef"=w555:T4)  [unwired: 8 in, 1 out]
          }
        }
      }
      n111 = while {
        tunnel: [w689] -> w509
        tunnel: w529 -> [w689]
        tunnel: [w682] -> w506
        tunnel: w527 -> [w682]
        tunnel: [w681] -> w505
        tunnel: w525 -> [w681]
        tunnel: w522 -> [w679]
        tunnel: [w678] -> w504
        tunnel: w519 -> [w677]
        tunnel: [w677] -> w507
        i -> [w684]
        stop <- w685 stop-if-true
        # "1/2 Sec."
        # "Lift Kit Up"
        n112 = Increment(x=w684) -> (x+1=w686:i32)
        n113 = global write "Robot Global Data.vi" "Gyro Reset"(TRUE) -> ()
        n114 = Wait (ms)(milliseconds to wait=u32 25) -> ()  [unwired: 1 out]
        n115 = Greater Or Equal?(x=w686, y=20) -> (x >= y?=w685:bool)
        n116 = call-poly <vilib>:"WPI_SolenoidSet.vi"("Value"=WPI_SolenoidValue."Forward", "SolenoidDevRef"=w679) -> ("SolenoidDevRef"=w678:T4)  [unwired: 8 in, 1 out]
      }
      n117 = flat-sequence {
        tunnel: [w581] -> w491
        tunnel: [w579] -> w489
        tunnel: [w575] -> w487
        tunnel: [w574] -> w485
        tunnel: [w573] -> w483
        tunnel: [u32 500 ("milliseconds to wait")] -> w481
        tunnel: w509 -> [w582]
        tunnel: w507 -> [w580]
        tunnel: w506 -> [w578]
        tunnel: w505 -> [w577]
        tunnel: w504 -> [w576]
        tunnel: w491 -> [w605]
        tunnel: [w605] -> w490
        tunnel: w489 -> [w604]
        tunnel: [w604] -> w488
        tunnel: w487 -> [w603]
        tunnel: [w603] -> w486
        tunnel: w485 -> [w602]
        tunnel: [w602] -> w484
        tunnel: w483 -> [w601]
        tunnel: [w601] -> w482
        tunnel: w481 -> [w600]
        tunnel: w490 -> [w607]
        tunnel: [w606] -> w480
        tunnel: w488 -> [w609]
        tunnel: [w608] -> w479
        tunnel: w486 -> [w611]
        tunnel: [w610] -> w478
        tunnel: w484 -> [w615]
        tunnel: [w613] -> w477
        tunnel: w482 -> [w614]
        tunnel: [w612] -> w476
        tunnel: w480 -> [w636]
        tunnel: [w636] -> w475
        tunnel: w479 -> [w635]
        tunnel: [w631] -> w474
        tunnel: w478 -> [w634]
        tunnel: [w634] -> w473
        tunnel: w477 -> [w633]
        tunnel: [w633] -> w472
        tunnel: w476 -> [w632]
        tunnel: [w632] -> w471
        tunnel: w475 -> [w643]
        tunnel: [w643] -> w470
        tunnel: w474 -> [w642]
        tunnel: [w638] -> w469
        tunnel: w473 -> [w641]
        tunnel: [w641] -> w468
        tunnel: w472 -> [w640]
        tunnel: [w640] -> w467
        tunnel: w471 -> [w639]
        tunnel: [w639] -> w466
        tunnel: w470 -> [w650]
        tunnel: [w650] -> w465
        tunnel: w469 -> [w649]
        tunnel: [w645] -> w463
        tunnel: w468 -> [w648]
        tunnel: [w648] -> w461
        tunnel: w467 -> [w647]
        tunnel: [w647] -> w459
        tunnel: w466 -> [w646]
        tunnel: [w646] -> w457
        tunnel: w465 -> [w658]
        tunnel: [w658] -> w464
        tunnel: w463 -> [w657]
        tunnel: [w653] -> w462
        tunnel: w461 -> [w656]
        tunnel: [w656] -> w460
        tunnel: w459 -> [w655]
        tunnel: [w655] -> w458
        tunnel: w457 -> [w654]
        tunnel: [w654] -> w456
        tunnel: [u32 5000 ("milliseconds to wait")] -> w455
        tunnel: [w660] -> w502
        tunnel: [w661] -> w503
        tunnel: [w662] -> w451
        tunnel: [w663] -> w454
        tunnel: [w664] -> w508
        tunnel: w464 -> [w664]
        tunnel: w462 -> [w663]
        tunnel: w460 -> [w662]
        tunnel: w458 -> [w661]
        tunnel: w456 -> [w660]
        tunnel: w455 -> [w659]
        frame #0 {
          n118 = while {
            tunnel: [w586] -> w581
            tunnel: w582 -> [w599]
            tunnel: [w583] -> w579
            tunnel: w580 -> [w583]
            tunnel: w578 -> [w598]
            tunnel: w577 -> [w597]
            tunnel: [w594] -> w575
            tunnel: w576 -> [w594]
            tunnel: [w593] -> w574
            tunnel: [w592] -> w573
            i -> [w588]
            stop <- w587 stop-if-true
            # "Drive Reverse To Brake."
            # "Shooting Motors Reverse 1 Sec."
            n119 = Increment(x=w588) -> (x+1=w590:i32)
            n120 = call <vilib>:"WPI_MotorControlSetOutput.vi"("Output"=0.5, "MotorControlDevRef"=w598) -> ("MotorControlDevRef"=w593:T7)  [unwired: 7 in, 2 out]
            n121 = Wait (ms)(milliseconds to wait=u32 25) -> ()  [unwired: 1 out]
            n122 = call <vilib>:"WPI_MotorControlSetOutput.vi"("Output"=-0.5, "MotorControlDevRef"=w597) -> ("MotorControlDevRef"=w592:T7)  [unwired: 7 in, 2 out]
            n123 = call <vilib>:"WPI_RobotDriveTankDrive.vi"("Right axis value"=0.05, "Left axis value"=0.05, "RobotDriveDevRef"=w599) -> ("RobotDriveDevRef"=w586:T6)  [unwired: 6 in, 2 out]
            n124 = Greater Or Equal?(x=w590, y=10) -> (x >= y?=w587:bool)
          }
        }
        frame #1 {
          # "Wait 1/2\nSec."
          n125 = Wait (ms)(milliseconds to wait=w600) -> ()  [unwired: 1 out]
        }
        frame #2 {
          n126 = while {
            tunnel: w615 -> [w629]
            tunnel: w614 -> [w628]
            tunnel: [w620] -> w613
            tunnel: [w619] -> w612
            tunnel: [w618] -> w610
            tunnel: w611 -> [w618]
            tunnel: [w617] -> w608
            tunnel: w609 -> [w617]
            tunnel: [w616] -> w606
            tunnel: w607 -> [w616]
            i -> [w624]
            stop <- w621 stop-if-true
            # "1/4 Sec."
            # "Shooting Motors Forward 20%."
            n127 = Increment(x=w624) -> (x+1=w623:i32)
            n128 = call <vilib>:"WPI_MotorControlSetOutput.vi"("Output"=0.2, "MotorControlDevRef"=w628) -> ("MotorControlDevRef"=w619:T7)  [unwired: 7 in, 2 out]
            n129 = call <vilib>:"WPI_MotorControlSetOutput.vi"("Output"=-0.2, "MotorControlDevRef"=w629) -> ("MotorControlDevRef"=w620:T7)  [unwired: 7 in, 2 out]
            n130 = Wait (ms)(milliseconds to wait=u32 10) -> ()  [unwired: 1 out]
            n131 = Greater Or Equal?(x=w623, y=25) -> (x >= y?=w621:bool)
          }
        }
        frame #3 {
          # "Up"
          n132 = call-poly <vilib>:"WPI_SolenoidSet.vi"("Value"=WPI_SolenoidValue."Reverse", "SolenoidDevRef"=w635) -> ("SolenoidDevRef"=w631:T4)  [unwired: 8 in, 1 out]
        }
        frame #4 {
          # "Down"
          n133 = call-poly <vilib>:"WPI_SolenoidSet.vi"("Value"=WPI_SolenoidValue."Forward", "SolenoidDevRef"=w642) -> ("SolenoidDevRef"=w638:T4)  [unwired: 8 in, 1 out]
        }
        frame #5 {
          # "Up"
          n134 = call-poly <vilib>:"WPI_SolenoidSet.vi"("Value"=WPI_SolenoidValue."Reverse", "SolenoidDevRef"=w649) -> ("SolenoidDevRef"=w645:T4)  [unwired: 8 in, 1 out]
        }
        frame #6 {
          # "Down"
          n135 = call-poly <vilib>:"WPI_SolenoidSet.vi"("Value"=WPI_SolenoidValue."Forward", "SolenoidDevRef"=w657) -> ("SolenoidDevRef"=w653:T4)  [unwired: 8 in, 1 out]
        }
        frame #7 {
          n136 = Wait (ms)(milliseconds to wait=w659) -> ()  [unwired: 1 out]
        }
      }
      n137 = while {
        tunnel: w508 -> [w732]
        tunnel: w503 -> [w728]
        tunnel: [w728] -> w511
        tunnel: [w727] -> w510
        tunnel: w502 -> [w727]
        tunnel: [w726] -> w513
        tunnel: [w725] -> w512
        tunnel: w451 -> [w725]
        tunnel: [w720] -> w453
        tunnel: w454 -> [w720]
        i -> [w723]
        stop <- w721 stop-if-true
        # "Turn Right 0.325 Sec."
        n138 = Increment(x=w723) -> (x+1=w724:i32)
        n139 = Wait (ms)(milliseconds to wait=u32 25) -> ()  [unwired: 1 out]
        n140 = call <vilib>:"WPI_RobotDriveTankDrive.vi"("Right axis value"=0.75, "Left axis value"=-0.75, "RobotDriveDevRef"=w732) -> ("RobotDriveDevRef"=w726:T6)  [unwired: 6 in, 2 out]
        n141 = Greater Or Equal?(x=w724, y=13) -> (x >= y?=w721:bool)
      }
      n142 = while {
        tunnel: [w712] -> w531
        tunnel: [w711] -> w530
        tunnel: w511 -> [w710]
        tunnel: w510 -> [w709]
        tunnel: [w708] -> w524
        tunnel: w513 -> [w708]
        tunnel: [w707] -> w521
        tunnel: w512 -> [w707]
        tunnel: [w706] -> w452
        tunnel: w453 -> [w706]
        i -> [w713]
        stop <- w714 stop-if-true
        # "Shooting Motors 97% for 1.25 Sec."
        n143 = Wait (ms)(milliseconds to wait=u32 25) -> ()  [unwired: 1 out]
        n144 = call <vilib>:"WPI_MotorControlSetOutput.vi"("Output"=0.97, "MotorControlDevRef"=w709) -> ("MotorControlDevRef"=w711:T7)  [unwired: 7 in, 2 out]
        n145 = call <vilib>:"WPI_MotorControlSetOutput.vi"("Output"=-0.97, "MotorControlDevRef"=w710) -> ("MotorControlDevRef"=w712:T7)  [unwired: 7 in, 2 out]
        n146 = Increment(x=w713) -> (x+1=w716:i32)
        n147 = Greater Or Equal?(x=w716, y=50) -> (x >= y?=w714:bool)
      }
      n148 = while {
        tunnel: w531 -> [w698]
        tunnel: w530 -> [w697]
        tunnel: [w695] -> w514
        tunnel: w524 -> [w695]
        tunnel: [w694] -> w515
        tunnel: w521 -> [w694]
        tunnel: [w693] -> w518
        tunnel: [w692] -> w516
        tunnel: [w691] -> w517
        tunnel: w452 -> [w690]
        i -> [w699]
        stop <- w700 stop-if-true
        # "1.25 Sec."
        # "Shooting Flippers Up"
        # "Shooting Motors Continue at 97%."
        n149 = Increment(x=w699) -> (x+1=w702:i32)
        n150 = Wait (ms)(milliseconds to wait=u32 25) -> ()  [unwired: 1 out]
        n151 = call <vilib>:"WPI_MotorControlSetOutput.vi"("Output"=0.97, "MotorControlDevRef"=w697) -> ("MotorControlDevRef"=w691:T7)  [unwired: 7 in, 2 out]
        n152 = call <vilib>:"WPI_MotorControlSetOutput.vi"("Output"=-0.97, "MotorControlDevRef"=w698) -> ("MotorControlDevRef"=w692:T7)  [unwired: 7 in, 2 out]
        n153 = Greater Or Equal?(x=w702, y=50) -> (x >= y?=w700:bool)
        n154 = call-poly <vilib>:"WPI_SolenoidSet.vi"("Value"=WPI_SolenoidValue."Reverse", "SolenoidDevRef"=w690) -> ("SolenoidDevRef"=w693:T4)  [unwired: 8 in, 1 out]
      }
      n155 = while {
        tunnel: w518 -> [w674]
        tunnel: w517 -> [w673]
        tunnel: w516 -> [w670]
        tunnel: w515 -> [w671]
        tunnel: w514 -> [w672]
        tunnel: [w673] -> w492
        tunnel: [w672] -> w495
        tunnel: [w671] -> w494
        tunnel: [w670] -> w493
        tunnel: [w669] -> w496
        i -> [w665]
        stop <- w666 stop-if-true
        # "1/2 Sec."
        # "Shooting Flippers Down"
        n156 = Increment(x=w665) -> (x+1=w667:i32)
        n157 = Wait (ms)(milliseconds to wait=u32 25) -> ()  [unwired: 1 out]
        n158 = Greater Or Equal?(x=w667, y=20) -> (x >= y?=w666:bool)
        n159 = call-poly <vilib>:"WPI_SolenoidSet.vi"("Value"=WPI_SolenoidValue."Forward", "SolenoidDevRef"=w674) -> ("SolenoidDevRef"=w669:T4)  [unwired: 8 in, 1 out]
      }
      n160 = while {
        tunnel: [w544] -> _
        tunnel: w496 -> [w544]
        tunnel: [w543] -> _
        tunnel: w495 -> [w543]
        tunnel: [w538] -> _
        tunnel: w494 -> [w542]
        tunnel: [w541] -> _
        tunnel: w493 -> [w541]
        tunnel: [w540] -> _
        tunnel: w492 -> [w540]
        i -> [w536]
        stop <- w534 stop-if-true
        # "1/2 Sec."
        # "Total Time: 14.075 Seconds."
        # "Lift-Kit Down"
        n161 = Increment(x=w536) -> (x+1=w535:i32)
        n162 = Wait (ms)(milliseconds to wait=u32 25) -> ()  [unwired: 1 out]
        n163 = Greater Or Equal?(x=w535, y=20) -> (x >= y?=w534:bool)
        n164 = call-poly <vilib>:"WPI_SolenoidSet.vi"("Value"=WPI_SolenoidValue."Reverse", "SolenoidDevRef"=w542) -> ("SolenoidDevRef"=w538:T4)  [unwired: 8 in, 1 out]
      }
    }
    frame "Drift Testing" {
      n165 = call <vilib>:"WPI_RobotDriveRefNum Registry Get.vi"("refnum name"="Left and Right Motors") -> ("RobotDriveDevRef"=w814:T6)  [unwired: 9 in, 1 out]
      n166 = call <vilib>:"WPI_MotorControlRefNum Registry Get.vi"("refnum name"="Top Motor") -> ("MotorControlDevRef"=w810:T7)  [unwired: 9 in, 1 out]
      n167 = call <vilib>:"WPI_MotorControlRefNum Registry Get.vi"("refnum name"="Bottom Motor") -> ("MotorControlDevRef"=w808:T7)  [unwired: 9 in, 1 out]
      n168 = call <vilib>:"WPI_SolenoidRefNum Registry Get.vi"("refnum name"="Lift Kit") -> ("SolenoidDevRef"=w805:T4)  [unwired: 9 in, 1 out]
      n169 = call <vilib>:"WPI_SolenoidRefNum Registry Get.vi"("refnum name"="Punch") -> ("SolenoidDevRef"=w802:T4)  [unwired: 9 in, 1 out]
      n170 = flat-sequence {
        tunnel: [w832] -> w801
        tunnel: [w833] -> w804
        tunnel: [w834] -> w807
        tunnel: [w835] -> w809
        tunnel: [w836] -> w811
        tunnel: w802 -> [w827]
        tunnel: w805 -> [w828]
        tunnel: w808 -> [w829]
        tunnel: w810 -> [w830]
        tunnel: w814 -> [w831]
        frame #0 {
          n171 = while {
            tunnel: w831 -> [w853]
            tunnel: [w846] -> w836
            tunnel: w830 -> [w844]
            tunnel: [w844] -> w835
            tunnel: w829 -> [w843]
            tunnel: [w843] -> w834
            tunnel: w828 -> [w842]
            tunnel: [w841] -> w833
            tunnel: [w837] -> w832
            tunnel: w827 -> [w838]
            i -> [w847]
            stop <- w848 stop-if-true
            # "Lift-Kit Down, Flippers Down."
            # "Drive Forward 2.5 Sec."
            n172 = Increment(x=w847) -> (x+1=w850:i32)
            n173 = call <vilib>:"WPI_RobotDriveTankDrive.vi"("Right axis value"=-0.6, "Left axis value"=-0.55, "RobotDriveDevRef"=w853) -> ("RobotDriveDevRef"=w846:T6)  [unwired: 6 in, 2 out]
            n174 = Wait (ms)(milliseconds to wait=u32 25) -> ()  [unwired: 1 out]
            n175 = Greater Or Equal?(x=w850, y=100) -> (x >= y?=w848:bool)
            n176 = call-poly <vilib>:"WPI_SolenoidSet.vi"("Value"=WPI_SolenoidValue."Reverse", "SolenoidDevRef"=w842) -> ("SolenoidDevRef"=w841:T4)  [unwired: 8 in, 1 out]
            n177 = call-poly <vilib>:"WPI_SolenoidSet.vi"("Value"=WPI_SolenoidValue."Forward", "SolenoidDevRef"=w838) -> ("SolenoidDevRef"=w837:T4)  [unwired: 8 in, 1 out]
          }
        }
      }
      n178 = while {
        tunnel: [w971] -> w791
        tunnel: w811 -> [w971]
        tunnel: [w964] -> w788
        tunnel: w809 -> [w964]
        tunnel: [w963] -> w787
        tunnel: w807 -> [w963]
        tunnel: w804 -> [w961]
        tunnel: [w960] -> w786
        tunnel: w801 -> [w959]
        tunnel: [w959] -> w789
        i -> [w966]
        stop <- w967 stop-if-true
        # "1/2 Sec."
        # "Lift Kit Up"
        n179 = Increment(x=w966) -> (x+1=w968:i32)
        n180 = global write "Robot Global Data.vi" "Gyro Reset"(TRUE) -> ()
        n181 = Wait (ms)(milliseconds to wait=u32 25) -> ()  [unwired: 1 out]
        n182 = Greater Or Equal?(x=w968, y=20) -> (x >= y?=w967:bool)
        n183 = call-poly <vilib>:"WPI_SolenoidSet.vi"("Value"=WPI_SolenoidValue."Forward", "SolenoidDevRef"=w961) -> ("SolenoidDevRef"=w960:T4)  [unwired: 8 in, 1 out]
      }
      n184 = flat-sequence {
        tunnel: [w863] -> w773
        tunnel: [w861] -> w771
        tunnel: [w857] -> w769
        tunnel: [w856] -> w767
        tunnel: [w855] -> w765
        tunnel: [u32 500 ("milliseconds to wait")] -> w763
        tunnel: w791 -> [w864]
        tunnel: w789 -> [w862]
        tunnel: w788 -> [w860]
        tunnel: w787 -> [w859]
        tunnel: w786 -> [w858]
        tunnel: w773 -> [w887]
        tunnel: [w887] -> w772
        tunnel: w771 -> [w886]
        tunnel: [w886] -> w770
        tunnel: w769 -> [w885]
        tunnel: [w885] -> w768
        tunnel: w767 -> [w884]
        tunnel: [w884] -> w766
        tunnel: w765 -> [w883]
        tunnel: [w883] -> w764
        tunnel: w763 -> [w882]
        tunnel: w772 -> [w889]
        tunnel: [w888] -> w762
        tunnel: w770 -> [w891]
        tunnel: [w890] -> w761
        tunnel: w768 -> [w893]
        tunnel: [w892] -> w760
        tunnel: w766 -> [w897]
        tunnel: [w895] -> w759
        tunnel: w764 -> [w896]
        tunnel: [w894] -> w758
        tunnel: w762 -> [w918]
        tunnel: [w918] -> w757
        tunnel: w761 -> [w917]
        tunnel: [w913] -> w756
        tunnel: w760 -> [w916]
        tunnel: [w916] -> w755
        tunnel: w759 -> [w915]
        tunnel: [w915] -> w754
        tunnel: w758 -> [w914]
        tunnel: [w914] -> w753
        tunnel: w757 -> [w925]
        tunnel: [w925] -> w752
        tunnel: w756 -> [w924]
        tunnel: [w920] -> w751
        tunnel: w755 -> [w923]
        tunnel: [w923] -> w750
        tunnel: w754 -> [w922]
        tunnel: [w922] -> w749
        tunnel: w753 -> [w921]
        tunnel: [w921] -> w748
        tunnel: w752 -> [w932]
        tunnel: [w932] -> w747
        tunnel: w751 -> [w931]
        tunnel: [w927] -> w745
        tunnel: w750 -> [w930]
        tunnel: [w930] -> w743
        tunnel: w749 -> [w929]
        tunnel: [w929] -> w741
        tunnel: w748 -> [w928]
        tunnel: [w928] -> w739
        tunnel: w747 -> [w940]
        tunnel: [w940] -> w746
        tunnel: w745 -> [w939]
        tunnel: [w935] -> w744
        tunnel: w743 -> [w938]
        tunnel: [w938] -> w742
        tunnel: w741 -> [w937]
        tunnel: [w937] -> w740
        tunnel: w739 -> [w936]
        tunnel: [w936] -> w738
        tunnel: [u32 5000 ("milliseconds to wait")] -> w737
        tunnel: [w942] -> w784
        tunnel: [w943] -> w785
        tunnel: [w944] -> w733
        tunnel: [w945] -> w736
        tunnel: [w946] -> w790
        tunnel: w746 -> [w946]
        tunnel: w744 -> [w945]
        tunnel: w742 -> [w944]
        tunnel: w740 -> [w943]
        tunnel: w738 -> [w942]
        tunnel: w737 -> [w941]
        frame #0 {
          n185 = while {
            tunnel: [w868] -> w863
            tunnel: w864 -> [w881]
            tunnel: [w865] -> w861
            tunnel: w862 -> [w865]
            tunnel: w860 -> [w880]
            tunnel: w859 -> [w879]
            tunnel: [w876] -> w857
            tunnel: w858 -> [w876]
            tunnel: [w875] -> w856
            tunnel: [w874] -> w855
            i -> [w870]
            stop <- w869 stop-if-true
            # "Drive Reverse To Brake."
            # "Shooting Motors Reverse 1 Sec."
            n186 = Increment(x=w870) -> (x+1=w872:i32)
            n187 = call <vilib>:"WPI_MotorControlSetOutput.vi"("Output"=0.5, "MotorControlDevRef"=w880) -> ("MotorControlDevRef"=w875:T7)  [unwired: 7 in, 2 out]
            n188 = Wait (ms)(milliseconds to wait=u32 25) -> ()  [unwired: 1 out]
            n189 = call <vilib>:"WPI_MotorControlSetOutput.vi"("Output"=-0.5, "MotorControlDevRef"=w879) -> ("MotorControlDevRef"=w874:T7)  [unwired: 7 in, 2 out]
            n190 = call <vilib>:"WPI_RobotDriveTankDrive.vi"("Right axis value"=0.05, "Left axis value"=0.05, "RobotDriveDevRef"=w881) -> ("RobotDriveDevRef"=w868:T6)  [unwired: 6 in, 2 out]
            n191 = Greater Or Equal?(x=w872, y=10) -> (x >= y?=w869:bool)
          }
        }
        frame #1 {
          # "Wait 1/2\nSec."
          n192 = Wait (ms)(milliseconds to wait=w882) -> ()  [unwired: 1 out]
        }
        frame #2 {
          n193 = while {
            tunnel: w897 -> [w911]
            tunnel: w896 -> [w910]
            tunnel: [w902] -> w895
            tunnel: [w901] -> w894
            tunnel: [w900] -> w892
            tunnel: w893 -> [w900]
            tunnel: [w899] -> w890
            tunnel: w891 -> [w899]
            tunnel: [w898] -> w888
            tunnel: w889 -> [w898]
            i -> [w906]
            stop <- w903 stop-if-true
            # "1/4 Sec."
            # "Shooting Motors Forward 20%."
            n194 = Increment(x=w906) -> (x+1=w905:i32)
            n195 = call <vilib>:"WPI_MotorControlSetOutput.vi"("Output"=0.2, "MotorControlDevRef"=w910) -> ("MotorControlDevRef"=w901:T7)  [unwired: 7 in, 2 out]
            n196 = call <vilib>:"WPI_MotorControlSetOutput.vi"("Output"=-0.2, "MotorControlDevRef"=w911) -> ("MotorControlDevRef"=w902:T7)  [unwired: 7 in, 2 out]
            n197 = Wait (ms)(milliseconds to wait=u32 10) -> ()  [unwired: 1 out]
            n198 = Greater Or Equal?(x=w905, y=25) -> (x >= y?=w903:bool)
          }
        }
        frame #3 {
          # "Up"
          n199 = call-poly <vilib>:"WPI_SolenoidSet.vi"("Value"=WPI_SolenoidValue."Reverse", "SolenoidDevRef"=w917) -> ("SolenoidDevRef"=w913:T4)  [unwired: 8 in, 1 out]
        }
        frame #4 {
          # "Down"
          n200 = call-poly <vilib>:"WPI_SolenoidSet.vi"("Value"=WPI_SolenoidValue."Forward", "SolenoidDevRef"=w924) -> ("SolenoidDevRef"=w920:T4)  [unwired: 8 in, 1 out]
        }
        frame #5 {
          # "Up"
          n201 = call-poly <vilib>:"WPI_SolenoidSet.vi"("Value"=WPI_SolenoidValue."Reverse", "SolenoidDevRef"=w931) -> ("SolenoidDevRef"=w927:T4)  [unwired: 8 in, 1 out]
        }
        frame #6 {
          # "Down"
          n202 = call-poly <vilib>:"WPI_SolenoidSet.vi"("Value"=WPI_SolenoidValue."Forward", "SolenoidDevRef"=w939) -> ("SolenoidDevRef"=w935:T4)  [unwired: 8 in, 1 out]
        }
        frame #7 {
          n203 = Wait (ms)(milliseconds to wait=w941) -> ()  [unwired: 1 out]
        }
      }
      n204 = while {
        tunnel: w790 -> [w1014]
        tunnel: w785 -> [w1010]
        tunnel: [w1010] -> w793
        tunnel: [w1009] -> w792
        tunnel: w784 -> [w1009]
        tunnel: [w1008] -> w795
        tunnel: [w1007] -> w794
        tunnel: w733 -> [w1007]
        tunnel: [w1002] -> w735
        tunnel: w736 -> [w1002]
        i -> [w1005]
        stop <- w1003 stop-if-true
        # "Turn Right 0.325 Sec."
        n205 = Increment(x=w1005) -> (x+1=w1006:i32)
        n206 = Wait (ms)(milliseconds to wait=u32 25) -> ()  [unwired: 1 out]
        n207 = call <vilib>:"WPI_RobotDriveTankDrive.vi"("Right axis value"=0.75, "Left axis value"=-0.75, "RobotDriveDevRef"=w1014) -> ("RobotDriveDevRef"=w1008:T6)  [unwired: 6 in, 2 out]
        n208 = Greater Or Equal?(x=w1006, y=13) -> (x >= y?=w1003:bool)
      }
      n209 = while {
        tunnel: [w994] -> w813
        tunnel: [w993] -> w812
        tunnel: w793 -> [w992]
        tunnel: w792 -> [w991]
        tunnel: [w990] -> w806
        tunnel: w795 -> [w990]
        tunnel: [w989] -> w803
        tunnel: w794 -> [w989]
        tunnel: [w988] -> w734
        tunnel: w735 -> [w988]
        i -> [w995]
        stop <- w996 stop-if-true
        # "Shooting Motors 97% for 1.25 Sec."
        n210 = Wait (ms)(milliseconds to wait=u32 25) -> ()  [unwired: 1 out]
        n211 = call <vilib>:"WPI_MotorControlSetOutput.vi"("Output"=0.97, "MotorControlDevRef"=w991) -> ("MotorControlDevRef"=w993:T7)  [unwired: 7 in, 2 out]
        n212 = call <vilib>:"WPI_MotorControlSetOutput.vi"("Output"=-0.97, "MotorControlDevRef"=w992) -> ("MotorControlDevRef"=w994:T7)  [unwired: 7 in, 2 out]
        n213 = Increment(x=w995) -> (x+1=w998:i32)
        n214 = Greater Or Equal?(x=w998, y=50) -> (x >= y?=w996:bool)
      }
      n215 = while {
        tunnel: w813 -> [w980]
        tunnel: w812 -> [w979]
        tunnel: [w977] -> w796
        tunnel: w806 -> [w977]
        tunnel: [w976] -> w797
        tunnel: w803 -> [w976]
        tunnel: [w975] -> w800
        tunnel: [w974] -> w798
        tunnel: [w973] -> w799
        tunnel: w734 -> [w972]
        i -> [w981]
        stop <- w982 stop-if-true
        # "1.25 Sec."
        # "Shooting Flippers Up"
        # "Shooting Motors Continue at 97%."
        n216 = Increment(x=w981) -> (x+1=w984:i32)
        n217 = Wait (ms)(milliseconds to wait=u32 25) -> ()  [unwired: 1 out]
        n218 = call <vilib>:"WPI_MotorControlSetOutput.vi"("Output"=0.97, "MotorControlDevRef"=w979) -> ("MotorControlDevRef"=w973:T7)  [unwired: 7 in, 2 out]
        n219 = call <vilib>:"WPI_MotorControlSetOutput.vi"("Output"=-0.97, "MotorControlDevRef"=w980) -> ("MotorControlDevRef"=w974:T7)  [unwired: 7 in, 2 out]
        n220 = Greater Or Equal?(x=w984, y=50) -> (x >= y?=w982:bool)
        n221 = call-poly <vilib>:"WPI_SolenoidSet.vi"("Value"=WPI_SolenoidValue."Reverse", "SolenoidDevRef"=w972) -> ("SolenoidDevRef"=w975:T4)  [unwired: 8 in, 1 out]
      }
      n222 = while {
        tunnel: w800 -> [w956]
        tunnel: w799 -> [w955]
        tunnel: w798 -> [w952]
        tunnel: w797 -> [w953]
        tunnel: w796 -> [w954]
        tunnel: [w955] -> w774
        tunnel: [w954] -> w777
        tunnel: [w953] -> w776
        tunnel: [w952] -> w775
        tunnel: [w951] -> w778
        i -> [w947]
        stop <- w948 stop-if-true
        # "1/2 Sec."
        # "Shooting Flippers Down"
        n223 = Increment(x=w947) -> (x+1=w949:i32)
        n224 = Wait (ms)(milliseconds to wait=u32 25) -> ()  [unwired: 1 out]
        n225 = Greater Or Equal?(x=w949, y=20) -> (x >= y?=w948:bool)
        n226 = call-poly <vilib>:"WPI_SolenoidSet.vi"("Value"=WPI_SolenoidValue."Forward", "SolenoidDevRef"=w956) -> ("SolenoidDevRef"=w951:T4)  [unwired: 8 in, 1 out]
      }
      n227 = while {
        tunnel: [w826] -> _
        tunnel: w778 -> [w826]
        tunnel: [w825] -> _
        tunnel: w777 -> [w825]
        tunnel: [w820] -> _
        tunnel: w776 -> [w824]
        tunnel: [w823] -> _
        tunnel: w775 -> [w823]
        tunnel: [w822] -> _
        tunnel: w774 -> [w822]
        i -> [w818]
        stop <- w816 stop-if-true
        # "1/2 Sec."
        # "Total Time: 14.075 Seconds."
        # "Lift-Kit Down"
        n228 = Increment(x=w818) -> (x+1=w817:i32)
        n229 = Wait (ms)(milliseconds to wait=u32 25) -> ()  [unwired: 1 out]
        n230 = Greater Or Equal?(x=w817, y=20) -> (x >= y?=w816:bool)
        n231 = call-poly <vilib>:"WPI_SolenoidSet.vi"("Value"=WPI_SolenoidValue."Reverse", "SolenoidDevRef"=w824) -> ("SolenoidDevRef"=w820:T4)  [unwired: 8 in, 1 out]
      }
    }
    frame "Low Bar Shot (Gyro)" {
      n232 = call <vilib>:"WPI_RobotDriveRefNum Registry Get.vi"("refnum name"="Left and Right Motors") -> ("RobotDriveDevRef"=w1096:T6)  [unwired: 9 in, 1 out]
      n233 = call <vilib>:"WPI_MotorControlRefNum Registry Get.vi"("refnum name"="Top Motor") -> ("MotorControlDevRef"=w1092:T7)  [unwired: 9 in, 1 out]
      n234 = call <vilib>:"WPI_MotorControlRefNum Registry Get.vi"("refnum name"="Bottom Motor") -> ("MotorControlDevRef"=w1090:T7)  [unwired: 9 in, 1 out]
      n235 = call <vilib>:"WPI_SolenoidRefNum Registry Get.vi"("refnum name"="Lift Kit") -> ("SolenoidDevRef"=w1087:T4)  [unwired: 9 in, 1 out]
      n236 = call <vilib>:"WPI_SolenoidRefNum Registry Get.vi"("refnum name"="Punch") -> ("SolenoidDevRef"=w1084:T4)  [unwired: 9 in, 1 out]
      n237 = flat-sequence {
        tunnel: [w1114] -> w1083
        tunnel: [w1115] -> w1086
        tunnel: [w1116] -> w1089
        tunnel: [w1117] -> w1091
        tunnel: [w1118] -> w1093
        tunnel: w1084 -> [w1109]
        tunnel: w1087 -> [w1110]
        tunnel: w1090 -> [w1111]
        tunnel: w1092 -> [w1112]
        tunnel: w1096 -> [w1113]
        frame #0 {
          n238 = while {
            tunnel: w1113 -> [w1135]
            tunnel: [w1128] -> w1118
            tunnel: w1112 -> [w1126]
            tunnel: [w1126] -> w1117
            tunnel: w1111 -> [w1125]
            tunnel: [w1125] -> w1116
            tunnel: w1110 -> [w1124]
            tunnel: [w1123] -> w1115
            tunnel: [w1119] -> w1114
            tunnel: w1109 -> [w1120]
            i -> [w1129]
            stop <- w1130 stop-if-true
            # "Lift-Kit Down, Flippers Down."
            # "Drive Forward 2 Sec."
            n239 = Increment(x=w1129) -> (x+1=w1132:i32)
            n240 = call <vilib>:"WPI_RobotDriveTankDrive.vi"("Right axis value"=-0.6, "Left axis value"=-0.6, "RobotDriveDevRef"=w1135) -> ("RobotDriveDevRef"=w1128:T6)  [unwired: 6 in, 2 out]
            n241 = Wait (ms)(milliseconds to wait=u32 25) -> ()  [unwired: 1 out]
            n242 = Greater Or Equal?(x=w1132, y=80) -> (x >= y?=w1130:bool)
            n243 = call-poly <vilib>:"WPI_SolenoidSet.vi"("Value"=WPI_SolenoidValue."Reverse", "SolenoidDevRef"=w1124) -> ("SolenoidDevRef"=w1123:T4)  [unwired: 8 in, 1 out]
            n244 = call-poly <vilib>:"WPI_SolenoidSet.vi"("Value"=WPI_SolenoidValue."Forward", "SolenoidDevRef"=w1120) -> ("SolenoidDevRef"=w1119:T4)  [unwired: 8 in, 1 out]
          }
        }
      }
      n245 = while {
        tunnel: [w1254] -> w1073
        tunnel: w1093 -> [w1254]
        tunnel: [w1247] -> w1070
        tunnel: w1091 -> [w1247]
        tunnel: [w1246] -> w1069
        tunnel: w1089 -> [w1246]
        tunnel: w1086 -> [w1244]
        tunnel: [w1243] -> w1068
        tunnel: w1083 -> [w1242]
        tunnel: [w1242] -> w1071
        i -> [w1249]
        stop <- w1250 stop-if-true
        # "1/2 Sec."
        # "Lift Kit Up"
        n246 = Increment(x=w1249) -> (x+1=w1251:i32)
        n247 = global write "Robot Global Data.vi" "Gyro Reset"(TRUE) -> ()
        n248 = Wait (ms)(milliseconds to wait=u32 25) -> ()  [unwired: 1 out]
        n249 = Greater Or Equal?(x=w1251, y=20) -> (x >= y?=w1250:bool)
        n250 = call-poly <vilib>:"WPI_SolenoidSet.vi"("Value"=WPI_SolenoidValue."Forward", "SolenoidDevRef"=w1244) -> ("SolenoidDevRef"=w1243:T4)  [unwired: 8 in, 1 out]
      }
      n251 = flat-sequence {
        tunnel: [w1145] -> w1055
        tunnel: [w1143] -> w1053
        tunnel: [w1139] -> w1051
        tunnel: [w1138] -> w1049
        tunnel: [w1137] -> w1047
        tunnel: [u32 500 ("milliseconds to wait")] -> w1045
        tunnel: w1073 -> [w1146]
        tunnel: w1071 -> [w1144]
        tunnel: w1070 -> [w1142]
        tunnel: w1069 -> [w1141]
        tunnel: w1068 -> [w1140]
        tunnel: w1055 -> [w1169]
        tunnel: [w1169] -> w1054
        tunnel: w1053 -> [w1168]
        tunnel: [w1168] -> w1052
        tunnel: w1051 -> [w1167]
        tunnel: [w1167] -> w1050
        tunnel: w1049 -> [w1166]
        tunnel: [w1166] -> w1048
        tunnel: w1047 -> [w1165]
        tunnel: [w1165] -> w1046
        tunnel: w1045 -> [w1164]
        tunnel: w1054 -> [w1171]
        tunnel: [w1170] -> w1044
        tunnel: w1052 -> [w1173]
        tunnel: [w1172] -> w1043
        tunnel: w1050 -> [w1175]
        tunnel: [w1174] -> w1042
        tunnel: w1048 -> [w1179]
        tunnel: [w1177] -> w1041
        tunnel: w1046 -> [w1178]
        tunnel: [w1176] -> w1040
        tunnel: w1044 -> [w1201]
        tunnel: [w1201] -> w1039
        tunnel: w1043 -> [w1200]
        tunnel: [w1196] -> w1038
        tunnel: w1042 -> [w1199]
        tunnel: [w1199] -> w1037
        tunnel: w1041 -> [w1198]
        tunnel: [w1198] -> w1036
        tunnel: w1040 -> [w1197]
        tunnel: [w1197] -> w1035
        tunnel: w1039 -> [w1208]
        tunnel: [w1208] -> w1034
        tunnel: w1038 -> [w1207]
        tunnel: [w1203] -> w1033
        tunnel: w1037 -> [w1206]
        tunnel: [w1206] -> w1032
        tunnel: w1036 -> [w1205]
        tunnel: [w1205] -> w1031
        tunnel: w1035 -> [w1204]
        tunnel: [w1204] -> w1030
        tunnel: w1034 -> [w1215]
        tunnel: [w1215] -> w1029
        tunnel: w1033 -> [w1214]
        tunnel: [w1210] -> w1027
        tunnel: w1032 -> [w1213]
        tunnel: [w1213] -> w1025
        tunnel: w1031 -> [w1212]
        tunnel: [w1212] -> w1023
        tunnel: w1030 -> [w1211]
        tunnel: [w1211] -> w1021
        tunnel: w1029 -> [w1223]
        tunnel: [w1223] -> w1028
        tunnel: w1027 -> [w1222]
        tunnel: [w1218] -> w1026
        tunnel: w1025 -> [w1221]
        tunnel: [w1221] -> w1024
        tunnel: w1023 -> [w1220]
        tunnel: [w1220] -> w1022
        tunnel: w1021 -> [w1219]
        tunnel: [w1219] -> w1020
        tunnel: [u32 5000 ("milliseconds to wait")] -> w1019
        tunnel: [w1225] -> w1066
        tunnel: [w1226] -> w1067
        tunnel: [w1227] -> w1015
        tunnel: [w1228] -> w1018
        tunnel: [w1229] -> w1072
        tunnel: w1028 -> [w1229]
        tunnel: w1026 -> [w1228]
        tunnel: w1024 -> [w1227]
        tunnel: w1022 -> [w1226]
        tunnel: w1020 -> [w1225]
        tunnel: w1019 -> [w1224]
        frame #0 {
          n252 = while {
            tunnel: [w1150] -> w1145
            tunnel: w1146 -> [w1163]
            tunnel: [w1147] -> w1143
            tunnel: w1144 -> [w1147]
            tunnel: w1142 -> [w1162]
            tunnel: w1141 -> [w1161]
            tunnel: [w1158] -> w1139
            tunnel: w1140 -> [w1158]
            tunnel: [w1157] -> w1138
            tunnel: [w1156] -> w1137
            i -> [w1152]
            stop <- w1151 stop-if-true
            # "Drive Reverse To Brake."
            # "Shooting Motors Reverse 1 Sec."
            n253 = Increment(x=w1152) -> (x+1=w1154:i32)
            n254 = call <vilib>:"WPI_MotorControlSetOutput.vi"("Output"=0.5, "MotorControlDevRef"=w1162) -> ("MotorControlDevRef"=w1157:T7)  [unwired: 7 in, 2 out]
            n255 = Wait (ms)(milliseconds to wait=u32 25) -> ()  [unwired: 1 out]
            n256 = call <vilib>:"WPI_MotorControlSetOutput.vi"("Output"=-0.5, "MotorControlDevRef"=w1161) -> ("MotorControlDevRef"=w1156:T7)  [unwired: 7 in, 2 out]
            n257 = call <vilib>:"WPI_RobotDriveTankDrive.vi"("Right axis value"=0.05, "Left axis value"=0.05, "RobotDriveDevRef"=w1163) -> ("RobotDriveDevRef"=w1150:T6)  [unwired: 6 in, 2 out]
            n258 = Greater Or Equal?(x=w1154, y=10) -> (x >= y?=w1151:bool)
          }
        }
        frame #1 {
          # "Wait 1/2\nSec."
          n259 = Wait (ms)(milliseconds to wait=w1164) -> ()  [unwired: 1 out]
        }
        frame #2 {
          n260 = while {
            tunnel: w1179 -> [w1194]
            tunnel: w1178 -> [w1193]
            tunnel: [w1185] -> w1177
            tunnel: [w1184] -> w1176
            tunnel: [w1183] -> w1174
            tunnel: w1175 -> [w1183]
            tunnel: [w1182] -> w1172
            tunnel: w1173 -> [w1182]
            tunnel: [w1181] -> w1170
            tunnel: w1171 -> [w1181]
            i -> [w1189]
            stop <- w1186 stop-if-true
            # "1/4 Sec."
            # "Shooting Motors Forward 20%."
            n261 = Increment(x=w1189) -> (x+1=w1188:i32)
            n262 = call <vilib>:"WPI_MotorControlSetOutput.vi"("Output"=0.2, "MotorControlDevRef"=w1193) -> ("MotorControlDevRef"=w1184:T7)  [unwired: 7 in, 2 out]
            n263 = call <vilib>:"WPI_MotorControlSetOutput.vi"("Output"=-0.2, "MotorControlDevRef"=w1194) -> ("MotorControlDevRef"=w1185:T7)  [unwired: 7 in, 2 out]
            n264 = Wait (ms)(milliseconds to wait=u32 10) -> ()  [unwired: 1 out]
            n265 = global write "Robot Global Data.vi" "Gyro Reset"(TRUE ("Gyro Reset")) -> ()
            n266 = Greater Or Equal?(x=w1188, y=25) -> (x >= y?=w1186:bool)
          }
        }
        frame #3 {
          # "Up"
          n267 = call-poly <vilib>:"WPI_SolenoidSet.vi"("Value"=WPI_SolenoidValue."Reverse", "SolenoidDevRef"=w1200) -> ("SolenoidDevRef"=w1196:T4)  [unwired: 8 in, 1 out]
        }
        frame #4 {
          # "Down"
          n268 = call-poly <vilib>:"WPI_SolenoidSet.vi"("Value"=WPI_SolenoidValue."Forward", "SolenoidDevRef"=w1207) -> ("SolenoidDevRef"=w1203:T4)  [unwired: 8 in, 1 out]
        }
        frame #5 {
          # "Up"
          n269 = call-poly <vilib>:"WPI_SolenoidSet.vi"("Value"=WPI_SolenoidValue."Reverse", "SolenoidDevRef"=w1214) -> ("SolenoidDevRef"=w1210:T4)  [unwired: 8 in, 1 out]
        }
        frame #6 {
          # "Down"
          n270 = call-poly <vilib>:"WPI_SolenoidSet.vi"("Value"=WPI_SolenoidValue."Forward", "SolenoidDevRef"=w1222) -> ("SolenoidDevRef"=w1218:T4)  [unwired: 8 in, 1 out]
        }
        frame #7 {
          n271 = Wait (ms)(milliseconds to wait=w1224) -> ()  [unwired: 1 out]
        }
      }
      n272 = while {
        tunnel: w1072 -> [w1296]
        tunnel: w1067 -> [w1292]
        tunnel: [w1292] -> w1075
        tunnel: [w1291] -> w1074
        tunnel: w1066 -> [w1291]
        tunnel: [w1290] -> w1077
        tunnel: [w1289] -> w1076
        tunnel: w1015 -> [w1289]
        tunnel: [w1288] -> w1017
        tunnel: w1018 -> [w1288]
        stop <- w1285 stop-if-true
        # "Turn Right 40 Deg."
        n273 = Wait (ms)(milliseconds to wait=u32 25) -> ()  [unwired: 1 out]
        n274 = call <vilib>:"WPI_RobotDriveTankDrive.vi"("Right axis value"=0.75, "Left axis value"=-0.75, "RobotDriveDevRef"=w1296) -> ("RobotDriveDevRef"=w1290:T6)  [unwired: 6 in, 2 out]
        n275 = global read "Robot Global Data.vi" "Gyro angle"() -> (w1287:dbl)
        n276 = Greater Or Equal?(x=w1287, y=-40.0) -> (x >= y?=w1285:bool)
      }
      n277 = while {
        tunnel: [w1277] -> w1095
        tunnel: [w1276] -> w1094
        tunnel: w1075 -> [w1275]
        tunnel: w1074 -> [w1274]
        tunnel: [w1273] -> w1088
        tunnel: w1077 -> [w1273]
        tunnel: [w1272] -> w1085
        tunnel: w1076 -> [w1272]
        tunnel: [w1271] -> w1016
        tunnel: w1017 -> [w1271]
        i -> [w1278]
        stop <- w1279 stop-if-true
        # "Shooting Motors 97% for 1.25 Sec."
        n278 = Wait (ms)(milliseconds to wait=u32 25) -> ()  [unwired: 1 out]
        n279 = call <vilib>:"WPI_MotorControlSetOutput.vi"("Output"=0.97, "MotorControlDevRef"=w1274) -> ("MotorControlDevRef"=w1276:T7)  [unwired: 7 in, 2 out]
        n280 = call <vilib>:"WPI_MotorControlSetOutput.vi"("Output"=-0.97, "MotorControlDevRef"=w1275) -> ("MotorControlDevRef"=w1277:T7)  [unwired: 7 in, 2 out]
        n281 = Increment(x=w1278) -> (x+1=w1281:i32)
        n282 = Greater Or Equal?(x=w1281, y=50) -> (x >= y?=w1279:bool)
      }
      n283 = while {
        tunnel: w1095 -> [w1263]
        tunnel: w1094 -> [w1262]
        tunnel: [w1260] -> w1078
        tunnel: w1088 -> [w1260]
        tunnel: [w1259] -> w1079
        tunnel: w1085 -> [w1259]
        tunnel: [w1258] -> w1082
        tunnel: [w1257] -> w1080
        tunnel: [w1256] -> w1081
        tunnel: w1016 -> [w1255]
        i -> [w1264]
        stop <- w1265 stop-if-true
        # "1.25 Sec."
        # "Shooting Flippers Up"
        # "Shooting Motors Continue at 97%."
        n284 = Increment(x=w1264) -> (x+1=w1267:i32)
        n285 = Wait (ms)(milliseconds to wait=u32 25) -> ()  [unwired: 1 out]
        n286 = call <vilib>:"WPI_MotorControlSetOutput.vi"("Output"=0.97, "MotorControlDevRef"=w1262) -> ("MotorControlDevRef"=w1256:T7)  [unwired: 7 in, 2 out]
        n287 = call <vilib>:"WPI_MotorControlSetOutput.vi"("Output"=-0.97, "MotorControlDevRef"=w1263) -> ("MotorControlDevRef"=w1257:T7)  [unwired: 7 in, 2 out]
        n288 = Greater Or Equal?(x=w1267, y=50) -> (x >= y?=w1265:bool)
        n289 = call-poly <vilib>:"WPI_SolenoidSet.vi"("Value"=WPI_SolenoidValue."Reverse", "SolenoidDevRef"=w1255) -> ("SolenoidDevRef"=w1258:T4)  [unwired: 8 in, 1 out]
      }
      n290 = while {
        tunnel: w1082 -> [w1239]
        tunnel: w1081 -> [w1238]
        tunnel: w1080 -> [w1235]
        tunnel: w1079 -> [w1236]
        tunnel: w1078 -> [w1237]
        tunnel: [w1238] -> w1056
        tunnel: [w1237] -> w1059
        tunnel: [w1236] -> w1058
        tunnel: [w1235] -> w1057
        tunnel: [w1234] -> w1060
        i -> [w1230]
        stop <- w1231 stop-if-true
        # "1/2 Sec."
        # "Shooting Flippers Down"
        n291 = Increment(x=w1230) -> (x+1=w1232:i32)
        n292 = Wait (ms)(milliseconds to wait=u32 25) -> ()  [unwired: 1 out]
        n293 = Greater Or Equal?(x=w1232, y=20) -> (x >= y?=w1231:bool)
        n294 = call-poly <vilib>:"WPI_SolenoidSet.vi"("Value"=WPI_SolenoidValue."Forward", "SolenoidDevRef"=w1239) -> ("SolenoidDevRef"=w1234:T4)  [unwired: 8 in, 1 out]
      }
      n295 = while {
        tunnel: [w1108] -> _
        tunnel: w1060 -> [w1108]
        tunnel: [w1107] -> _
        tunnel: w1059 -> [w1107]
        tunnel: [w1102] -> _
        tunnel: w1058 -> [w1106]
        tunnel: [w1105] -> _
        tunnel: w1057 -> [w1105]
        tunnel: [w1104] -> _
        tunnel: w1056 -> [w1104]
        i -> [w1100]
        stop <- w1098 stop-if-true
        # "1/2 Sec."
        # "Total Time: 14.075 Seconds."
        # "Lift-Kit Down"
        n296 = Increment(x=w1100) -> (x+1=w1099:i32)
        n297 = Wait (ms)(milliseconds to wait=u32 25) -> ()  [unwired: 1 out]
        n298 = Greater Or Equal?(x=w1099, y=20) -> (x >= y?=w1098:bool)
        n299 = call-poly <vilib>:"WPI_SolenoidSet.vi"("Value"=WPI_SolenoidValue."Reverse", "SolenoidDevRef"=w1106) -> ("SolenoidDevRef"=w1102:T4)  [unwired: 8 in, 1 out]
      }
    }
    frame "Low-Bar Low Goal" {
      n300 = call <vilib>:"WPI_RobotDriveRefNum Registry Get.vi"("refnum name"="Left and Right Motors") -> ("RobotDriveDevRef"=w1358:T6)  [unwired: 9 in, 1 out]
      n301 = call <vilib>:"WPI_MotorControlRefNum Registry Get.vi"("refnum name"="Top Motor") -> ("MotorControlDevRef"=w1354:T7)  [unwired: 9 in, 1 out]
      n302 = call <vilib>:"WPI_MotorControlRefNum Registry Get.vi"("refnum name"="Bottom Motor") -> ("MotorControlDevRef"=w1352:T7)  [unwired: 9 in, 1 out]
      n303 = call <vilib>:"WPI_SolenoidRefNum Registry Get.vi"("refnum name"="Lift Kit") -> ("SolenoidDevRef"=w1349:T4)  [unwired: 9 in, 1 out]
      n304 = call <vilib>:"WPI_SolenoidRefNum Registry Get.vi"("refnum name"="Punch") -> ("SolenoidDevRef"=w1346:T4)  [unwired: 9 in, 1 out]
      n305 = flat-sequence {
        tunnel: [w1376] -> w1345
        tunnel: [w1377] -> w1348
        tunnel: [w1378] -> w1351
        tunnel: [w1379] -> w1353
        tunnel: [w1380] -> w1355
        tunnel: w1346 -> [w1371]
        tunnel: w1349 -> [w1372]
        tunnel: w1352 -> [w1373]
        tunnel: w1354 -> [w1374]
        tunnel: w1358 -> [w1375]
        frame #0 {
          n306 = while {
            tunnel: w1375 -> [w1397]
            tunnel: [w1390] -> w1380
            tunnel: w1374 -> [w1388]
            tunnel: [w1388] -> w1379
            tunnel: w1373 -> [w1387]
            tunnel: [w1387] -> w1378
            tunnel: w1372 -> [w1386]
            tunnel: [w1385] -> w1377
            tunnel: [w1381] -> w1376
            tunnel: w1371 -> [w1382]
            i -> [w1391]
            stop <- w1392 stop-if-true
            # "Lift-Kit Down, Flippers Down."
            # "Drive Forward 3 Sec."
            n307 = Increment(x=w1391) -> (x+1=w1394:i32)
            n308 = call <vilib>:"WPI_RobotDriveTankDrive.vi"("Right axis value"=-0.6, "Left axis value"=-0.6, "RobotDriveDevRef"=w1397) -> ("RobotDriveDevRef"=w1390:T6)  [unwired: 6 in, 2 out]
            n309 = Wait (ms)(milliseconds to wait=u32 25) -> ()  [unwired: 1 out]
            n310 = Greater Or Equal?(x=w1394, y=120) -> (x >= y?=w1392:bool)
            n311 = call-poly <vilib>:"WPI_SolenoidSet.vi"("Value"=WPI_SolenoidValue."Reverse", "SolenoidDevRef"=w1386) -> ("SolenoidDevRef"=w1385:T4)  [unwired: 8 in, 1 out]
            n312 = call-poly <vilib>:"WPI_SolenoidSet.vi"("Value"=WPI_SolenoidValue."Forward", "SolenoidDevRef"=w1382) -> ("SolenoidDevRef"=w1381:T4)  [unwired: 8 in, 1 out]
          }
        }
      }
      n313 = while {
        tunnel: [w1487] -> w1333
        tunnel: w1355 -> [w1487]
        tunnel: [w1480] -> w1330
        tunnel: w1353 -> [w1480]
        tunnel: [w1479] -> w1329
        tunnel: w1351 -> [w1479]
        tunnel: w1348 -> [w1477]
        tunnel: [w1476] -> w1328
        tunnel: w1345 -> [w1475]
        tunnel: [w1475] -> w1331
        i -> [w1482]
        stop <- w1483 stop-if-true
        # "1/2 Sec."
        # "Lift Kit Up"
        n314 = Increment(x=w1482) -> (x+1=w1484:i32)
        n315 = global write "Robot Global Data.vi" "Gyro Reset"(TRUE) -> ()
        n316 = Wait (ms)(milliseconds to wait=u32 25) -> ()  [unwired: 1 out]
        n317 = Greater Or Equal?(x=w1484, y=20) -> (x >= y?=w1483:bool)
        n318 = call-poly <vilib>:"WPI_SolenoidSet.vi"("Value"=WPI_SolenoidValue."Forward", "SolenoidDevRef"=w1477) -> ("SolenoidDevRef"=w1476:T4)  [unwired: 8 in, 1 out]
      }
      n319 = flat-sequence {
        tunnel: [w1407] -> w1309
        tunnel: [w1405] -> w1307
        tunnel: [w1401] -> w1305
        tunnel: [w1400] -> w1303
        tunnel: [w1399] -> w1301
        tunnel: w1333 -> [w1408]
        tunnel: w1331 -> [w1406]
        tunnel: w1330 -> [w1404]
        tunnel: w1329 -> [w1403]
        tunnel: w1328 -> [w1402]
        tunnel: [u32 500 ("milliseconds to wait")] -> w1299
        tunnel: w1309 -> [w1431]
        tunnel: [w1431] -> w1308
        tunnel: w1307 -> [w1430]
        tunnel: [w1430] -> w1306
        tunnel: w1305 -> [w1429]
        tunnel: [w1429] -> w1304
        tunnel: w1303 -> [w1428]
        tunnel: [w1428] -> w1302
        tunnel: w1301 -> [w1427]
        tunnel: [w1427] -> w1300
        tunnel: w1299 -> [w1426]
        tunnel: w1308 -> [w1437]
        tunnel: [w1436] -> w1320
        tunnel: w1306 -> [w1433]
        tunnel: [w1432] -> w1319
        tunnel: w1304 -> [w1435]
        tunnel: [w1434] -> w1318
        tunnel: w1302 -> [w1442]
        tunnel: [w1440] -> w1317
        tunnel: w1300 -> [w1441]
        tunnel: [w1439] -> w1316
        tunnel: [u32 5000 ("milliseconds to wait")] -> w1315
        tunnel: [w1458] -> w1326
        tunnel: [w1459] -> w1327
        tunnel: [w1460] -> w1297
        tunnel: [w1461] -> w1298
        tunnel: [w1462] -> w1332
        tunnel: w1320 -> [w1462]
        tunnel: w1319 -> [w1461]
        tunnel: w1318 -> [w1460]
        tunnel: w1317 -> [w1459]
        tunnel: w1316 -> [w1458]
        tunnel: w1315 -> [w1457]
        frame #0 {
          n320 = while {
            tunnel: [w1412] -> w1407
            tunnel: w1408 -> [w1425]
            tunnel: [w1409] -> w1405
            tunnel: w1406 -> [w1409]
            tunnel: w1404 -> [w1424]
            tunnel: w1403 -> [w1423]
            tunnel: [w1420] -> w1401
            tunnel: w1402 -> [w1420]
            tunnel: [w1419] -> w1400
            tunnel: [w1418] -> w1399
            i -> [w1414]
            stop <- w1413 stop-if-true
            # "Drive Reverse To Brake."
            # "Shooting Motors Reverse 1 Sec."
            n321 = Increment(x=w1414) -> (x+1=w1416:i32)
            n322 = call <vilib>:"WPI_MotorControlSetOutput.vi"("Output"=0.5, "MotorControlDevRef"=w1424) -> ("MotorControlDevRef"=w1419:T7)  [unwired: 7 in, 2 out]
            n323 = Wait (ms)(milliseconds to wait=u32 25) -> ()  [unwired: 1 out]
            n324 = call <vilib>:"WPI_MotorControlSetOutput.vi"("Output"=-0.5, "MotorControlDevRef"=w1423) -> ("MotorControlDevRef"=w1418:T7)  [unwired: 7 in, 2 out]
            n325 = call <vilib>:"WPI_RobotDriveTankDrive.vi"("Right axis value"=0.05, "Left axis value"=0.05, "RobotDriveDevRef"=w1425) -> ("RobotDriveDevRef"=w1412:T6)  [unwired: 6 in, 2 out]
            n326 = Greater Or Equal?(x=w1416, y=40) -> (x >= y?=w1413:bool)
          }
        }
        frame #1 {
          # "Wait 1/2\nSec."
          n327 = Wait (ms)(milliseconds to wait=w1426) -> ()  [unwired: 1 out]
        }
        frame #2 {
          n328 = while {
            tunnel: w1442 -> [w1456]
            tunnel: w1441 -> [w1455]
            tunnel: [w1447] -> w1440
            tunnel: [w1446] -> w1439
            tunnel: [w1445] -> w1436
            tunnel: w1437 -> [w1445]
            tunnel: [w1444] -> w1434
            tunnel: w1435 -> [w1444]
            tunnel: [w1443] -> w1432
            tunnel: w1433 -> [w1443]
            i -> [w1451]
            stop <- w1448 stop-if-true
            # "1/4 Sec."
            # "Shooting Motors Forward 20%."
            n329 = Increment(x=w1451) -> (x+1=w1450:i32)
            n330 = call <vilib>:"WPI_MotorControlSetOutput.vi"("Output"=0.2, "MotorControlDevRef"=w1455) -> ("MotorControlDevRef"=w1446:T7)  [unwired: 7 in, 2 out]
            n331 = call <vilib>:"WPI_MotorControlSetOutput.vi"("Output"=-0.2, "MotorControlDevRef"=w1456) -> ("MotorControlDevRef"=w1447:T7)  [unwired: 7 in, 2 out]
            n332 = Wait (ms)(milliseconds to wait=u32 10) -> ()  [unwired: 1 out]
            n333 = Greater Or Equal?(x=w1450, y=25) -> (x >= y?=w1448:bool)
          }
        }
        frame #3 {
          # "Wait 5 Sec."
          n334 = Wait (ms)(milliseconds to wait=w1457) -> ()  [unwired: 1 out]
        }
      }
      n335 = while {
        tunnel: w1332 -> [w1530]
        tunnel: w1327 -> [w1526]
        tunnel: [w1526] -> w1335
        tunnel: [w1525] -> w1334
        tunnel: w1326 -> [w1525]
        tunnel: [w1524] -> w1337
        tunnel: [w1523] -> w1336
        tunnel: w1297 -> [w1523]
        tunnel: [w1522] -> w1338
        tunnel: w1298 -> [w1522]
        i -> [w1520]
        stop <- w1518 stop-if-true
        # "Turn Right 0.325 Sec."
        n336 = Increment(x=w1520) -> (x+1=w1521:i32)
        n337 = Wait (ms)(milliseconds to wait=u32 25) -> ()  [unwired: 1 out]
        n338 = call <vilib>:"WPI_RobotDriveTankDrive.vi"("Right axis value"=0.75, "Left axis value"=-0.75, "RobotDriveDevRef"=w1530) -> ("RobotDriveDevRef"=w1524:T6)  [unwired: 6 in, 2 out]
        n339 = Greater Or Equal?(x=w1521, y=13) -> (x >= y?=w1518:bool)
      }
      n340 = while {
        tunnel: [w1510] -> w1357
        tunnel: [w1509] -> w1356
        tunnel: w1335 -> [w1508]
        tunnel: w1334 -> [w1507]
        tunnel: [w1506] -> w1350
        tunnel: w1337 -> [w1506]
        tunnel: [w1505] -> w1347
        tunnel: w1336 -> [w1505]
        tunnel: w1338 -> [w1504]
        tunnel: [w1504] -> w1344
        i -> [w1511]
        stop <- w1512 stop-if-true
        # "Shooting Motors 60% for 1.25 Sec."
        n341 = Wait (ms)(milliseconds to wait=u32 25) -> ()  [unwired: 1 out]
        n342 = call <vilib>:"WPI_MotorControlSetOutput.vi"("Output"=0.6, "MotorControlDevRef"=w1507) -> ("MotorControlDevRef"=w1509:T7)  [unwired: 7 in, 2 out]
        n343 = call <vilib>:"WPI_MotorControlSetOutput.vi"("Output"=-0.6, "MotorControlDevRef"=w1508) -> ("MotorControlDevRef"=w1510:T7)  [unwired: 7 in, 2 out]
        n344 = Increment(x=w1511) -> (x+1=w1514:i32)
        n345 = Greater Or Equal?(x=w1514, y=50) -> (x >= y?=w1512:bool)
      }
      n346 = while {
        tunnel: w1357 -> [w1496]
        tunnel: w1356 -> [w1495]
        tunnel: [w1493] -> w1339
        tunnel: w1350 -> [w1493]
        tunnel: [w1492] -> w1340
        tunnel: w1347 -> [w1492]
        tunnel: w1344 -> [w1491]
        tunnel: [w1490] -> w1343
        tunnel: [w1489] -> w1341
        tunnel: [w1488] -> w1342
        i -> [w1497]
        stop <- w1498 stop-if-true
        # "1.25 Sec."
        # "Shooting Flippers Up"
        # "Shooting Motors Continue at 60%."
        n347 = Increment(x=w1497) -> (x+1=w1500:i32)
        n348 = call <vilib>:"WPI_MotorControlSetOutput.vi"("Output"=0.6, "MotorControlDevRef"=w1495) -> ("MotorControlDevRef"=w1488:T7)  [unwired: 7 in, 2 out]
        n349 = call <vilib>:"WPI_MotorControlSetOutput.vi"("Output"=-0.6, "MotorControlDevRef"=w1496) -> ("MotorControlDevRef"=w1489:T7)  [unwired: 7 in, 2 out]
        n350 = Wait (ms)(milliseconds to wait=u32 25) -> ()  [unwired: 1 out]
        n351 = Greater Or Equal?(x=w1500, y=50) -> (x >= y?=w1498:bool)
        n352 = call-poly <vilib>:"WPI_SolenoidSet.vi"("Value"=WPI_SolenoidValue."Reverse", "SolenoidDevRef"=w1491) -> ("SolenoidDevRef"=w1490:T4)  [unwired: 8 in, 1 out]
      }
      n353 = while {
        tunnel: w1343 -> [w1472]
        tunnel: w1342 -> [w1471]
        tunnel: w1341 -> [w1468]
        tunnel: w1340 -> [w1469]
        tunnel: w1339 -> [w1470]
        tunnel: [w1471] -> w1310
        tunnel: [w1470] -> w1313
        tunnel: [w1469] -> w1312
        tunnel: [w1468] -> w1311
        tunnel: [w1467] -> w1314
        i -> [w1463]
        stop <- w1464 stop-if-true
        # "Shooting Flippers Down"
        n354 = Increment(x=w1463) -> (x+1=w1465:i32)
        n355 = Wait (ms)(milliseconds to wait=u32 25) -> ()  [unwired: 1 out]
        n356 = Greater Or Equal?(x=w1465, y=20) -> (x >= y?=w1464:bool)
        n357 = call-poly <vilib>:"WPI_SolenoidSet.vi"("Value"=WPI_SolenoidValue."Forward", "SolenoidDevRef"=w1472) -> ("SolenoidDevRef"=w1467:T4)  [unwired: 8 in, 1 out]
      }
      n358 = while {
        tunnel: [w1370] -> _
        tunnel: w1314 -> [w1370]
        tunnel: [w1369] -> _
        tunnel: w1313 -> [w1369]
        tunnel: [w1364] -> _
        tunnel: w1312 -> [w1368]
        tunnel: [w1367] -> _
        tunnel: w1311 -> [w1367]
        tunnel: [w1366] -> _
        tunnel: w1310 -> [w1366]
        i -> [w1362]
        stop <- w1360 stop-if-true
        # "Total Time: 14.075 Seconds."
        # "Lift-Kit Down"
        n359 = Increment(x=w1362) -> (x+1=w1361:i32)
        n360 = Wait (ms)(milliseconds to wait=u32 25) -> ()  [unwired: 1 out]
        n361 = Greater Or Equal?(x=w1361, y=20) -> (x >= y?=w1360:bool)
        n362 = call-poly <vilib>:"WPI_SolenoidSet.vi"("Value"=WPI_SolenoidValue."Reverse", "SolenoidDevRef"=w1368) -> ("SolenoidDevRef"=w1364:T4)  [unwired: 8 in, 1 out]
      }
    }
    frame "Low Bar Low Goal (Gyro)" {
      n363 = call <vilib>:"WPI_RobotDriveRefNum Registry Get.vi"("refnum name"="Left and Right Motors") -> ("RobotDriveDevRef"=w1592:T6)  [unwired: 9 in, 1 out]
      n364 = call <vilib>:"WPI_MotorControlRefNum Registry Get.vi"("refnum name"="Top Motor") -> ("MotorControlDevRef"=w1588:T7)  [unwired: 9 in, 1 out]
      n365 = call <vilib>:"WPI_MotorControlRefNum Registry Get.vi"("refnum name"="Bottom Motor") -> ("MotorControlDevRef"=w1586:T7)  [unwired: 9 in, 1 out]
      n366 = call <vilib>:"WPI_SolenoidRefNum Registry Get.vi"("refnum name"="Lift Kit") -> ("SolenoidDevRef"=w1583:T4)  [unwired: 9 in, 1 out]
      n367 = call <vilib>:"WPI_SolenoidRefNum Registry Get.vi"("refnum name"="Punch") -> ("SolenoidDevRef"=w1580:T4)  [unwired: 9 in, 1 out]
      n368 = flat-sequence {
        tunnel: [w1610] -> w1579
        tunnel: [w1611] -> w1582
        tunnel: [w1612] -> w1585
        tunnel: [w1613] -> w1587
        tunnel: [w1614] -> w1589
        tunnel: w1580 -> [w1605]
        tunnel: w1583 -> [w1606]
        tunnel: w1586 -> [w1607]
        tunnel: w1588 -> [w1608]
        tunnel: w1592 -> [w1609]
        frame #0 {
          n369 = while {
            tunnel: w1609 -> [w1631]
            tunnel: [w1624] -> w1614
            tunnel: w1608 -> [w1622]
            tunnel: [w1622] -> w1613
            tunnel: w1607 -> [w1621]
            tunnel: [w1621] -> w1612
            tunnel: w1606 -> [w1620]
            tunnel: [w1619] -> w1611
            tunnel: [w1615] -> w1610
            tunnel: w1605 -> [w1616]
            i -> [w1625]
            stop <- w1626 stop-if-true
            # "Lift-Kit Down, Flippers Down."
            # "Drive Forward 3 Sec."
            n370 = Increment(x=w1625) -> (x+1=w1628:i32)
            n371 = call <vilib>:"WPI_RobotDriveTankDrive.vi"("Right axis value"=-0.6, "Left axis value"=-0.6, "RobotDriveDevRef"=w1631) -> ("RobotDriveDevRef"=w1624:T6)  [unwired: 6 in, 2 out]
            n372 = Wait (ms)(milliseconds to wait=u32 25) -> ()  [unwired: 1 out]
            n373 = Greater Or Equal?(x=w1628, y=120) -> (x >= y?=w1626:bool)
            n374 = call-poly <vilib>:"WPI_SolenoidSet.vi"("Value"=WPI_SolenoidValue."Reverse", "SolenoidDevRef"=w1620) -> ("SolenoidDevRef"=w1619:T4)  [unwired: 8 in, 1 out]
            n375 = call-poly <vilib>:"WPI_SolenoidSet.vi"("Value"=WPI_SolenoidValue."Forward", "SolenoidDevRef"=w1616) -> ("SolenoidDevRef"=w1615:T4)  [unwired: 8 in, 1 out]
          }
        }
      }
      n376 = while {
        tunnel: [w1722] -> w1567
        tunnel: w1589 -> [w1722]
        tunnel: [w1715] -> w1564
        tunnel: w1587 -> [w1715]
        tunnel: [w1714] -> w1563
        tunnel: w1585 -> [w1714]
        tunnel: w1582 -> [w1712]
        tunnel: [w1711] -> w1562
        tunnel: w1579 -> [w1710]
        tunnel: [w1710] -> w1565
        i -> [w1717]
        stop <- w1718 stop-if-true
        # "1/2 Sec."
        # "Lift Kit Up"
        n377 = Increment(x=w1717) -> (x+1=w1719:i32)
        n378 = global write "Robot Global Data.vi" "Gyro Reset"(TRUE) -> ()
        n379 = Wait (ms)(milliseconds to wait=u32 25) -> ()  [unwired: 1 out]
        n380 = Greater Or Equal?(x=w1719, y=20) -> (x >= y?=w1718:bool)
        n381 = call-poly <vilib>:"WPI_SolenoidSet.vi"("Value"=WPI_SolenoidValue."Forward", "SolenoidDevRef"=w1712) -> ("SolenoidDevRef"=w1711:T4)  [unwired: 8 in, 1 out]
      }
      n382 = flat-sequence {
        tunnel: [w1641] -> w1543
        tunnel: [w1639] -> w1541
        tunnel: [w1635] -> w1539
        tunnel: [w1634] -> w1537
        tunnel: [w1633] -> w1535
        tunnel: w1567 -> [w1642]
        tunnel: w1565 -> [w1640]
        tunnel: w1564 -> [w1638]
        tunnel: w1563 -> [w1637]
        tunnel: w1562 -> [w1636]
        tunnel: [u32 500 ("milliseconds to wait")] -> w1533
        tunnel: w1543 -> [w1665]
        tunnel: [w1665] -> w1542
        tunnel: w1541 -> [w1664]
        tunnel: [w1664] -> w1540
        tunnel: w1539 -> [w1663]
        tunnel: [w1663] -> w1538
        tunnel: w1537 -> [w1662]
        tunnel: [w1662] -> w1536
        tunnel: w1535 -> [w1661]
        tunnel: [w1661] -> w1534
        tunnel: w1533 -> [w1660]
        tunnel: w1542 -> [w1671]
        tunnel: [w1670] -> w1554
        tunnel: w1540 -> [w1667]
        tunnel: [w1666] -> w1553
        tunnel: w1538 -> [w1669]
        tunnel: [w1668] -> w1552
        tunnel: w1536 -> [w1676]
        tunnel: [w1674] -> w1551
        tunnel: w1534 -> [w1675]
        tunnel: [w1673] -> w1550
        tunnel: [u32 5000 ("milliseconds to wait")] -> w1549
        tunnel: [w1693] -> w1560
        tunnel: [w1694] -> w1561
        tunnel: [w1695] -> w1531
        tunnel: [w1696] -> w1532
        tunnel: [w1697] -> w1566
        tunnel: w1554 -> [w1697]
        tunnel: w1553 -> [w1696]
        tunnel: w1552 -> [w1695]
        tunnel: w1551 -> [w1694]
        tunnel: w1550 -> [w1693]
        tunnel: w1549 -> [w1692]
        frame #0 {
          n383 = while {
            tunnel: [w1646] -> w1641
            tunnel: w1642 -> [w1659]
            tunnel: [w1643] -> w1639
            tunnel: w1640 -> [w1643]
            tunnel: w1638 -> [w1658]
            tunnel: w1637 -> [w1657]
            tunnel: [w1654] -> w1635
            tunnel: w1636 -> [w1654]
            tunnel: [w1653] -> w1634
            tunnel: [w1652] -> w1633
            i -> [w1648]
            stop <- w1647 stop-if-true
            # "Drive Reverse To Brake."
            # "Shooting Motors Reverse 1 Sec."
            n384 = Increment(x=w1648) -> (x+1=w1650:i32)
            n385 = call <vilib>:"WPI_MotorControlSetOutput.vi"("Output"=0.5, "MotorControlDevRef"=w1658) -> ("MotorControlDevRef"=w1653:T7)  [unwired: 7 in, 2 out]
            n386 = Wait (ms)(milliseconds to wait=u32 25) -> ()  [unwired: 1 out]
            n387 = call <vilib>:"WPI_MotorControlSetOutput.vi"("Output"=-0.5, "MotorControlDevRef"=w1657) -> ("MotorControlDevRef"=w1652:T7)  [unwired: 7 in, 2 out]
            n388 = call <vilib>:"WPI_RobotDriveTankDrive.vi"("Right axis value"=0.05, "Left axis value"=0.05, "RobotDriveDevRef"=w1659) -> ("RobotDriveDevRef"=w1646:T6)  [unwired: 6 in, 2 out]
            n389 = Greater Or Equal?(x=w1650, y=40) -> (x >= y?=w1647:bool)
          }
        }
        frame #1 {
          # "Wait 1/2\nSec."
          n390 = Wait (ms)(milliseconds to wait=w1660) -> ()  [unwired: 1 out]
        }
        frame #2 {
          n391 = while {
            tunnel: w1676 -> [w1691]
            tunnel: w1675 -> [w1690]
            tunnel: [w1682] -> w1674
            tunnel: [w1681] -> w1673
            tunnel: [w1680] -> w1670
            tunnel: w1671 -> [w1680]
            tunnel: [w1679] -> w1668
            tunnel: w1669 -> [w1679]
            tunnel: [w1678] -> w1666
            tunnel: w1667 -> [w1678]
            i -> [w1686]
            stop <- w1683 stop-if-true
            # "1/4 Sec."
            # "Shooting Motors Forward 20%."
            n392 = Increment(x=w1686) -> (x+1=w1685:i32)
            n393 = call <vilib>:"WPI_MotorControlSetOutput.vi"("Output"=0.2, "MotorControlDevRef"=w1690) -> ("MotorControlDevRef"=w1681:T7)  [unwired: 7 in, 2 out]
            n394 = call <vilib>:"WPI_MotorControlSetOutput.vi"("Output"=-0.2, "MotorControlDevRef"=w1691) -> ("MotorControlDevRef"=w1682:T7)  [unwired: 7 in, 2 out]
            n395 = Wait (ms)(milliseconds to wait=u32 10) -> ()  [unwired: 1 out]
            n396 = global write "Robot Global Data.vi" "Gyro Reset"(TRUE ("Gyro Reset")) -> ()
            n397 = Greater Or Equal?(x=w1685, y=25) -> (x >= y?=w1683:bool)
          }
        }
        frame #3 {
          # "Wait 5 Sec."
          n398 = Wait (ms)(milliseconds to wait=w1692) -> ()  [unwired: 1 out]
        }
      }
      n399 = while {
        tunnel: w1566 -> [w1764]
        tunnel: w1561 -> [w1760]
        tunnel: [w1760] -> w1569
        tunnel: [w1759] -> w1568
        tunnel: w1560 -> [w1759]
        tunnel: [w1758] -> w1571
        tunnel: [w1757] -> w1570
        tunnel: w1531 -> [w1757]
        tunnel: [w1756] -> w1572
        tunnel: w1532 -> [w1756]
        stop <- w1753 stop-if-true
        # "Turn Right 30 Deg."
        n400 = Wait (ms)(milliseconds to wait=u32 25) -> ()  [unwired: 1 out]
        n401 = call <vilib>:"WPI_RobotDriveTankDrive.vi"("Right axis value"=0.75, "Left axis value"=-0.75, "RobotDriveDevRef"=w1764) -> ("RobotDriveDevRef"=w1758:T6)  [unwired: 6 in, 2 out]
        n402 = global read "Robot Global Data.vi" "Gyro angle"() -> (w1755:dbl)
        n403 = Greater Or Equal?(x=w1755, y=-30.0) -> (x >= y?=w1753:bool)
      }
      n404 = while {
        tunnel: [w1745] -> w1591
        tunnel: [w1744] -> w1590
        tunnel: w1569 -> [w1743]
        tunnel: w1568 -> [w1742]
        tunnel: [w1741] -> w1584
        tunnel: w1571 -> [w1741]
        tunnel: [w1740] -> w1581
        tunnel: w1570 -> [w1740]
        tunnel: w1572 -> [w1739]
        tunnel: [w1739] -> w1578
        i -> [w1746]
        stop <- w1747 stop-if-true
        # "Shooting Motors 60% for 1.25 Sec."
        n405 = Wait (ms)(milliseconds to wait=u32 25) -> ()  [unwired: 1 out]
        n406 = call <vilib>:"WPI_MotorControlSetOutput.vi"("Output"=0.6, "MotorControlDevRef"=w1742) -> ("MotorControlDevRef"=w1744:T7)  [unwired: 7 in, 2 out]
        n407 = call <vilib>:"WPI_MotorControlSetOutput.vi"("Output"=-0.6, "MotorControlDevRef"=w1743) -> ("MotorControlDevRef"=w1745:T7)  [unwired: 7 in, 2 out]
        n408 = Increment(x=w1746) -> (x+1=w1749:i32)
        n409 = Greater Or Equal?(x=w1749, y=50) -> (x >= y?=w1747:bool)
      }
      n410 = while {
        tunnel: w1591 -> [w1731]
        tunnel: w1590 -> [w1730]
        tunnel: [w1728] -> w1573
        tunnel: w1584 -> [w1728]
        tunnel: [w1727] -> w1574
        tunnel: w1581 -> [w1727]
        tunnel: w1578 -> [w1726]
        tunnel: [w1725] -> w1577
        tunnel: [w1724] -> w1575
        tunnel: [w1723] -> w1576
        i -> [w1732]
        stop <- w1733 stop-if-true
        # "1.25 Sec."
        # "Shooting Flippers Up"
        # "Shooting Motors Continue at 60%."
        n411 = Increment(x=w1732) -> (x+1=w1735:i32)
        n412 = call <vilib>:"WPI_MotorControlSetOutput.vi"("Output"=0.6, "MotorControlDevRef"=w1730) -> ("MotorControlDevRef"=w1723:T7)  [unwired: 7 in, 2 out]
        n413 = call <vilib>:"WPI_MotorControlSetOutput.vi"("Output"=-0.6, "MotorControlDevRef"=w1731) -> ("MotorControlDevRef"=w1724:T7)  [unwired: 7 in, 2 out]
        n414 = Wait (ms)(milliseconds to wait=u32 25) -> ()  [unwired: 1 out]
        n415 = Greater Or Equal?(x=w1735, y=50) -> (x >= y?=w1733:bool)
        n416 = call-poly <vilib>:"WPI_SolenoidSet.vi"("Value"=WPI_SolenoidValue."Reverse", "SolenoidDevRef"=w1726) -> ("SolenoidDevRef"=w1725:T4)  [unwired: 8 in, 1 out]
      }
      n417 = while {
        tunnel: w1577 -> [w1707]
        tunnel: w1576 -> [w1706]
        tunnel: w1575 -> [w1703]
        tunnel: w1574 -> [w1704]
        tunnel: w1573 -> [w1705]
        tunnel: [w1706] -> w1544
        tunnel: [w1705] -> w1547
        tunnel: [w1704] -> w1546
        tunnel: [w1703] -> w1545
        tunnel: [w1702] -> w1548
        i -> [w1698]
        stop <- w1699 stop-if-true
        # "Shooting Flippers Down"
        n418 = Increment(x=w1698) -> (x+1=w1700:i32)
        n419 = Wait (ms)(milliseconds to wait=u32 25) -> ()  [unwired: 1 out]
        n420 = Greater Or Equal?(x=w1700, y=20) -> (x >= y?=w1699:bool)
        n421 = call-poly <vilib>:"WPI_SolenoidSet.vi"("Value"=WPI_SolenoidValue."Forward", "SolenoidDevRef"=w1707) -> ("SolenoidDevRef"=w1702:T4)  [unwired: 8 in, 1 out]
      }
      n422 = while {
        tunnel: [w1604] -> _
        tunnel: w1548 -> [w1604]
        tunnel: [w1603] -> _
        tunnel: w1547 -> [w1603]
        tunnel: [w1598] -> _
        tunnel: w1546 -> [w1602]
        tunnel: [w1601] -> _
        tunnel: w1545 -> [w1601]
        tunnel: [w1600] -> _
        tunnel: w1544 -> [w1600]
        i -> [w1596]
        stop <- w1594 stop-if-true
        # "Total Time: 14.075 Seconds."
        # "Lift-Kit Down"
        n423 = Increment(x=w1596) -> (x+1=w1595:i32)
        n424 = Wait (ms)(milliseconds to wait=u32 25) -> ()  [unwired: 1 out]
        n425 = Greater Or Equal?(x=w1595, y=20) -> (x >= y?=w1594:bool)
        n426 = call-poly <vilib>:"WPI_SolenoidSet.vi"("Value"=WPI_SolenoidValue."Reverse", "SolenoidDevRef"=w1602) -> ("SolenoidDevRef"=w1598:T4)  [unwired: 8 in, 1 out]
      }
    }
    frame "Rock Wall/Ramparts" {
      n427 = call <vilib>:"WPI_RobotDriveRefNum Registry Get.vi"("refnum name"="Left and Right Motors") -> ("RobotDriveDevRef"=w1783:T6)  [unwired: 9 in, 1 out]
      n428 = call <vilib>:"WPI_SolenoidRefNum Registry Get.vi"("refnum name"="Lift Kit") -> ("SolenoidDevRef"=w1780:T4)  [unwired: 9 in, 1 out]
      n429 = call <vilib>:"WPI_MotorControlRefNum Registry Get.vi"("refnum name"="Bottom Motor") -> ("MotorControlDevRef"=w1770:T7)  [unwired: 9 in, 1 out]
      n430 = call <vilib>:"WPI_MotorControlRefNum Registry Get.vi"("refnum name"="Top Motor") -> ("MotorControlDevRef"=w1774:T7)  [unwired: 9 in, 1 out]
      n431 = while {
        tunnel: w1783 -> [w1830]
        tunnel: [w1823] -> w1782
        tunnel: [w1822] -> w1779
        tunnel: w1780 -> [w1822]
        tunnel: [w1821] -> w1773
        tunnel: w1774 -> [w1821]
        tunnel: [w1820] -> w1769
        tunnel: w1770 -> [w1820]
        i -> [w1828]
        stop <- w1826 stop-if-true
        w1829 = -0.6 ("Left axis value")
        # "Drive Forward 60% 1 Sec."
        n432 = Increment(x=w1828) -> (x+1=w1827:i32)
        n433 = call <vilib>:"WPI_RobotDriveTankDrive.vi"("Right axis value"=w1829, "Left axis value"=w1829, "RobotDriveDevRef"=w1830) -> ("RobotDriveDevRef"=w1823:T6)  [unwired: 6 in, 2 out]
        n434 = Greater Or Equal?(x=w1827, y=40) -> (x >= y?=w1826:bool)
        n435 = Wait (ms)(milliseconds to wait=u32 25) -> ()  [unwired: 1 out]
      }
      n436 = while {
        tunnel: w1782 -> [w1819]
        tunnel: [w1817] -> w1777
        tunnel: [w1811] -> w1778
        tunnel: w1779 -> [w1811]
        tunnel: [w1810] -> w1772
        tunnel: w1773 -> [w1810]
        tunnel: [w1809] -> w1768
        tunnel: w1769 -> [w1809]
        i -> [w1815]
        stop <- w1813 stop-if-true
        w1818 = -0.9 ("Left axis value")
        # "Drive Forward 90% 1 Sec."
        n437 = Increment(x=w1815) -> (x+1=w1814:i32)
        n438 = call <vilib>:"WPI_RobotDriveTankDrive.vi"("Right axis value"=w1818, "Left axis value"=w1818, "RobotDriveDevRef"=w1819) -> ("RobotDriveDevRef"=w1817:T6)  [unwired: 6 in, 2 out]
        n439 = Wait (ms)(milliseconds to wait=u32 25) -> ()  [unwired: 1 out]
        n440 = Greater Or Equal?(x=w1814, y=40) -> (x >= y?=w1813:bool)
      }
      n441 = while {
        tunnel: [w1807] -> w1766
        tunnel: w1778 -> [w1808]
        tunnel: [w1800] -> w1765
        tunnel: w1777 -> [w1800]
        tunnel: [w1799] -> w1771
        tunnel: w1772 -> [w1799]
        tunnel: [w1798] -> w1767
        tunnel: w1768 -> [w1798]
        i -> [w1805]
        stop <- w1802 stop-if-true
        # "Lift Kit up 1/2 Sec."
        n442 = Increment(x=w1805) -> (x+1=w1804:i32)
        n443 = call-poly <vilib>:"WPI_SolenoidSet.vi"("Value"=WPI_SolenoidValue."Forward", "SolenoidDevRef"=w1808) -> ("SolenoidDevRef"=w1807:T4)  [unwired: 8 in, 1 out]
        n444 = Greater Or Equal?(x=w1804, y=20) -> (x >= y?=w1802:bool)
        n445 = Wait (ms)(milliseconds to wait=u32 25) -> ()  [unwired: 1 out]
      }
      n446 = while {
        tunnel: w1771 -> [w1795]
        tunnel: w1767 -> [w1794]
        tunnel: [w1788] -> _
        tunnel: w1766 -> [w1788]
        tunnel: [w1787] -> _
        tunnel: w1765 -> [w1787]
        tunnel: [w1786] -> _
        tunnel: [w1785] -> _
        i -> [w1792]
        stop <- w1789 stop-if-true
        # "Total Time: 3.5 Sec."
        # "Motors Reverse 1 Sec."
        n447 = Increment(x=w1792) -> (x+1=w1791:i32)
        n448 = call <vilib>:"WPI_MotorControlSetOutput.vi"("Output"=0.5, "MotorControlDevRef"=w1795) -> ("MotorControlDevRef"=w1786:T7)  [unwired: 7 in, 2 out]
        n449 = call <vilib>:"WPI_MotorControlSetOutput.vi"("Output"=-0.5, "MotorControlDevRef"=w1794) -> ("MotorControlDevRef"=w1785:T7)  [unwired: 7 in, 2 out]
        n450 = Greater Or Equal?(x=w1791, y=40) -> (x >= y?=w1789:bool)
        n451 = Wait (ms)(milliseconds to wait=u32 25) -> ()  [unwired: 1 out]
      }
    }
    frame "Moat/Rough Terrain" {
      n452 = call <vilib>:"WPI_RobotDriveRefNum Registry Get.vi"("refnum name"="Left and Right Motors") -> ("RobotDriveDevRef"=w1846:T6)  [unwired: 9 in, 1 out]
      n453 = call <vilib>:"WPI_SolenoidRefNum Registry Get.vi"("refnum name"="Lift Kit") -> ("SolenoidDevRef"=w1841:T4)  [unwired: 9 in, 1 out]
      n454 = call <vilib>:"WPI_MotorControlRefNum Registry Get.vi"("refnum name"="Top Motor") -> ("MotorControlDevRef"=w1840:T7)  [unwired: 9 in, 1 out]
      n455 = call <vilib>:"WPI_MotorControlRefNum Registry Get.vi"("refnum name"="Bottom Motor") -> ("MotorControlDevRef"=w1839:T7)  [unwired: 9 in, 1 out]
      n456 = while {
        tunnel: w1846 -> [w1881]
        tunnel: [w1880] -> w1836
        tunnel: [w1873] -> w1838
        tunnel: w1841 -> [w1873]
        tunnel: [w1872] -> w1835
        tunnel: w1840 -> [w1872]
        tunnel: [w1871] -> w1834
        tunnel: w1839 -> [w1871]
        i -> [w1877]
        stop <- w1874 stop-if-true
        w1878 = -0.75 ("Right axis value")
        # "Drive Forward 75% 2 Sec."
        n457 = Wait (ms)(milliseconds to wait=u32 25) -> ()  [unwired: 1 out]
        n458 = call <vilib>:"WPI_RobotDriveTankDrive.vi"("Right axis value"=w1878, "Left axis value"=w1878, "RobotDriveDevRef"=w1881) -> ("RobotDriveDevRef"=w1880:T6)  [unwired: 6 in, 2 out]
        n459 = Increment(x=w1877) -> (x+1=w1876:i32)
        n460 = Greater Or Equal?(x=w1876, y=120) -> (x >= y?=w1874:bool)
      }
      n461 = while {
        tunnel: w1838 -> [w1870]
        tunnel: [w1868] -> w1837
        tunnel: [w1863] -> w1831
        tunnel: w1836 -> [w1863]
        tunnel: [w1862] -> w1833
        tunnel: w1835 -> [w1862]
        tunnel: [w1861] -> w1832
        tunnel: w1834 -> [w1861]
        i -> [w1867]
        stop <- w1864 stop-if-true
        # "Lift Kit up 1 Sec."
        n462 = Increment(x=w1867) -> (x+1=w1866:i32)
        n463 = call-poly <vilib>:"WPI_SolenoidSet.vi"("Value"=WPI_SolenoidValue."Forward", "SolenoidDevRef"=w1870) -> ("SolenoidDevRef"=w1868:T4)  [unwired: 8 in, 1 out]
        n464 = Greater Or Equal?(x=w1866, y=40) -> (x >= y?=w1864:bool)
        n465 = Wait (ms)(milliseconds to wait=u32 25) -> ()  [unwired: 1 out]
      }
      n466 = while {
        tunnel: [w1859] -> _
        tunnel: w1837 -> [w1859]
        tunnel: w1833 -> [w1858]
        tunnel: w1832 -> [w1857]
        tunnel: [w1854] -> _
        tunnel: [w1853] -> _
        tunnel: [w1852] -> _
        tunnel: w1831 -> [w1852]
        i -> [w1850]
        stop <- w1847 stop-if-true
        # "Total Time: 4 Sec."
        # "Shooters Reverse 1 Sec."
        n467 = call <vilib>:"WPI_MotorControlSetOutput.vi"("Output"=-0.5, "MotorControlDevRef"=w1857) -> ("MotorControlDevRef"=w1854:T7)  [unwired: 7 in, 2 out]
        n468 = call <vilib>:"WPI_MotorControlSetOutput.vi"("Output"=0.5, "MotorControlDevRef"=w1858) -> ("MotorControlDevRef"=w1853:T7)  [unwired: 7 in, 2 out]
        n469 = Increment(x=w1850) -> (x+1=w1849:i32)
        n470 = Greater Or Equal?(x=w1849, y=40) -> (x >= y?=w1847:bool)
        n471 = Wait (ms)(milliseconds to wait=u32 25) -> ()  [unwired: 1 out]
      }
    }
    frame "Approach Defense", Default {
      n472 = call <vilib>:"WPI_RobotDriveRefNum Registry Get.vi"("refnum name"="Left and Right Motors") -> ("RobotDriveDevRef"=w1897:T6)  [unwired: 9 in, 1 out]
      n473 = call <vilib>:"WPI_MotorControlRefNum Registry Get.vi"("refnum name"="Top Motor") -> ("MotorControlDevRef"=w1890:T7)  [unwired: 9 in, 1 out]
      n474 = call <vilib>:"WPI_MotorControlRefNum Registry Get.vi"("refnum name"="Bottom Motor") -> ("MotorControlDevRef"=w1891:T7)  [unwired: 9 in, 1 out]
      n475 = call <vilib>:"WPI_SolenoidRefNum Registry Get.vi"("refnum name"="Lift Kit") -> ("SolenoidDevRef"=w1892:T4)  [unwired: 9 in, 1 out]
      n476 = while {
        tunnel: w1897 -> [w1932]
        tunnel: [w1931] -> w1886
        tunnel: [w1924] -> w1889
        tunnel: w1892 -> [w1924]
        tunnel: [w1923] -> w1888
        tunnel: w1891 -> [w1923]
        tunnel: [w1922] -> w1887
        tunnel: w1890 -> [w1922]
        i -> [w1928]
        stop <- w1925 stop-if-true
        w1930 = -0.45 ("Left axis value")
        # "Drive Forward 3.5 Sec."
        n477 = Increment(x=w1928) -> (x+1=w1927:i32)
        n478 = call <vilib>:"WPI_RobotDriveTankDrive.vi"("Right axis value"=w1930, "Left axis value"=w1930, "RobotDriveDevRef"=w1932) -> ("RobotDriveDevRef"=w1931:T6)  [unwired: 6 in, 2 out]
        n479 = Wait (ms)(milliseconds to wait=u32 25) -> ()  [unwired: 1 out]
        n480 = Greater Or Equal?(x=w1927, y=140) -> (x >= y?=w1925:bool)
      }
      n481 = while {
        tunnel: [w1917] -> w1885
        tunnel: w1889 -> [w1921]
        tunnel: [w1920] -> w1884
        tunnel: w1888 -> [w1920]
        tunnel: [w1919] -> w1883
        tunnel: w1887 -> [w1919]
        tunnel: [w1918] -> w1882
        tunnel: w1886 -> [w1918]
        i -> [w1914]
        stop <- w1911 stop-if-true
        # "Lift Kit Up 1 Sec."
        n482 = call-poly <vilib>:"WPI_SolenoidSet.vi"("Value"=WPI_SolenoidValue."Forward", "SolenoidDevRef"=w1921) -> ("SolenoidDevRef"=w1917:T4)  [unwired: 8 in, 1 out]
        n483 = Increment(x=w1914) -> (x+1=w1913:i32)
        n484 = Greater Or Equal?(x=w1913, y=40) -> (x >= y?=w1911:bool)
        n485 = Wait (ms)(milliseconds to wait=u32 25) -> ()  [unwired: 1 out]
      }
      n486 = while {
        tunnel: [w1910] -> _
        tunnel: w1885 -> [w1910]
        tunnel: [w1906] -> _
        tunnel: w1884 -> [w1909]
        tunnel: [w1904] -> _
        tunnel: w1883 -> [w1908]
        tunnel: [w1907] -> _
        tunnel: w1882 -> [w1907]
        i -> [w1902]
        stop <- w1899 stop-if-true
        # "Total Time: 4 Sec."
        # "Shooters Reverse 1 Sec."
        n487 = Increment(x=w1902) -> (x+1=w1901:i32)
        n488 = call <vilib>:"WPI_MotorControlSetOutput.vi"("Output"=0.5, "MotorControlDevRef"=w1909) -> ("MotorControlDevRef"=w1906:T7)  [unwired: 7 in, 2 out]
        n489 = call <vilib>:"WPI_MotorControlSetOutput.vi"("Output"=-0.5, "MotorControlDevRef"=w1908) -> ("MotorControlDevRef"=w1904:T7)  [unwired: 7 in, 2 out]
        n490 = Greater Or Equal?(x=w1901, y=40) -> (x >= y?=w1899:bool)
        n491 = Wait (ms)(milliseconds to wait=u32 25) -> ()  [unwired: 1 out]
      }
    }
    frame "Spy Bot Shot" {
      n492 = call <vilib>:"WPI_MotorControlRefNum Registry Get.vi"("refnum name"="Top Motor") -> ("MotorControlDevRef"=w1957:T7)  [unwired: 9 in, 1 out]
      n493 = call <vilib>:"WPI_MotorControlRefNum Registry Get.vi"("refnum name"="Bottom Motor") -> ("MotorControlDevRef"=w1955:T7)  [unwired: 9 in, 1 out]
      n494 = call <vilib>:"WPI_SolenoidRefNum Registry Get.vi"("refnum name"="Punch") -> ("SolenoidDevRef"=w1959:T4)  [unwired: 9 in, 1 out]
      n495 = call <vilib>:"WPI_SolenoidRefNum Registry Get.vi"("refnum name"="Lift Kit") -> ("SolenoidDevRef"=w1961:T4)  [unwired: 9 in, 1 out]
      n496 = while {
        tunnel: w1961 -> [w2066]
        tunnel: [w2065] -> w1960
        tunnel: [w2055] -> w1958
        tunnel: w1959 -> [w2064]
        tunnel: [w2063] -> w1956
        tunnel: w1957 -> [w2063]
        tunnel: [w2062] -> w1954
        tunnel: w1955 -> [w2062]
        i -> [w2059]
        stop <- w2056 stop-if-true
        # "Lift Kit Up 1 Sec."
        n497 = Increment(x=w2059) -> (x+1=w2058:i32)
        n498 = Wait (ms)(milliseconds to wait=u32 25) -> ()  [unwired: 1 out]
        n499 = Greater Or Equal?(x=w2058, y=40) -> (x >= y?=w2056:bool)
        n500 = call-poly <vilib>:"WPI_SolenoidSet.vi"("Value"=WPI_SolenoidValue."Forward", "SolenoidDevRef"=w2064) -> ("SolenoidDevRef"=w2055:T4)  [unwired: 8 in, 1 out]
        n501 = call-poly <vilib>:"WPI_SolenoidSet.vi"("Value"=WPI_SolenoidValue."Forward", "SolenoidDevRef"=w2066) -> ("SolenoidDevRef"=w2065:T4)  [unwired: 8 in, 1 out]
      }
      n502 = while {
        tunnel: [w2053] -> w1952
        tunnel: w1960 -> [w2053]
        tunnel: [w2052] -> w1953
        tunnel: w1958 -> [w2052]
        tunnel: [w2049] -> w1951
        tunnel: w1956 -> [w2051]
        tunnel: [w2047] -> w1950
        tunnel: w1954 -> [w2050]
        i -> [w2044]
        stop <- w2041 stop-if-true
        # "1 Sec."
        # "Reverse Shooter To Drop Ball."
        n503 = Increment(x=w2044) -> (x+1=w2043:i32)
        n504 = call <vilib>:"WPI_MotorControlSetOutput.vi"("Output"=0.4, "MotorControlDevRef"=w2051) -> ("MotorControlDevRef"=w2049:T7)  [unwired: 7 in, 2 out]
        n505 = call <vilib>:"WPI_MotorControlSetOutput.vi"("Output"=-0.4, "MotorControlDevRef"=w2050) -> ("MotorControlDevRef"=w2047:T7)  [unwired: 7 in, 2 out]
        n506 = Wait (ms)(milliseconds to wait=u32 25) -> ()  [unwired: 1 out]
        n507 = Greater Or Equal?(x=w2043, y=40) -> (x >= y?=w2041:bool)
      }
      n508 = flat-sequence {
        tunnel: [w2019] -> w1949
        tunnel: [w2018] -> w1948
        tunnel: [w2017] -> w1947
        tunnel: [w2016] -> w1946
        tunnel: w1950 -> [w2016]
        tunnel: w1951 -> [w2017]
        tunnel: w1952 -> [w2018]
        tunnel: w1953 -> [w2019]
        tunnel: u32 6000 ("milliseconds to wait") -> [w2015]
        tunnel: w1949 -> [w2027]
        tunnel: w1948 -> [w2026]
        tunnel: w1947 -> [w2025]
        tunnel: w1946 -> [w2024]
        tunnel: [w2023] -> w1945
        tunnel: [w2022] -> w1944
        tunnel: [w2021] -> w1943
        tunnel: [w2020] -> w1942
        frame #0 {
          # "Wait 6\nSec."
          n509 = Wait (ms)(milliseconds to wait=w2015) -> ()  [unwired: 1 out]
        }
        frame #1 {
          n510 = while {
            tunnel: [w2040] -> w2023
            tunnel: w2027 -> [w2040]
            tunnel: [w2039] -> w2022
            tunnel: w2026 -> [w2039]
            tunnel: [w2036] -> w2021
            tunnel: w2025 -> [w2038]
            tunnel: [w2034] -> w2020
            tunnel: w2024 -> [w2037]
            i -> [w2031]
            stop <- w2028 stop-if-true
            # "Spool Up Shooter 2 Sec."
            n511 = Increment(x=w2031) -> (x+1=w2030:i32)
            n512 = Wait (ms)(milliseconds to wait=u32 25) -> ()  [unwired: 1 out]
            n513 = call <vilib>:"WPI_MotorControlSetOutput.vi"("Output"=0.97, "MotorControlDevRef"=w2037) -> ("MotorControlDevRef"=w2034:T7)  [unwired: 7 in, 2 out]
            n514 = call <vilib>:"WPI_MotorControlSetOutput.vi"("Output"=-0.97, "MotorControlDevRef"=w2038) -> ("MotorControlDevRef"=w2036:T7)  [unwired: 7 in, 2 out]
            n515 = Greater Or Equal?(x=w2030, y=80) -> (x >= y?=w2028:bool)
          }
        }
      }
      n516 = while {
        tunnel: [w2001] -> w1938
        tunnel: w1945 -> [w2014]
        tunnel: [w2013] -> w1939
        tunnel: w1944 -> [w2013]
        tunnel: [w2003] -> w1940
        tunnel: w1943 -> [w2012]
        tunnel: [w2005] -> w1941
        tunnel: w1942 -> [w2011]
        i -> [w2009]
        stop <- w2006 stop-if-true
        # "Shoot Ball 1 Sec."
        n517 = Increment(x=w2009) -> (x+1=w2008:i32)
        n518 = Wait (ms)(milliseconds to wait=u32 25) -> ()  [unwired: 1 out]
        n519 = call <vilib>:"WPI_MotorControlSetOutput.vi"("Output"=0.97, "MotorControlDevRef"=w2011) -> ("MotorControlDevRef"=w2005:T7)  [unwired: 7 in, 2 out]
        n520 = Greater Or Equal?(x=w2008, y=40) -> (x >= y?=w2006:bool)
        n521 = call-poly <vilib>:"WPI_SolenoidSet.vi"("Value"=WPI_SolenoidValue."Reverse", "SolenoidDevRef"=w2014) -> ("SolenoidDevRef"=w2001:T4)  [unwired: 8 in, 1 out]
        n522 = call <vilib>:"WPI_MotorControlSetOutput.vi"("Output"=-0.97, "MotorControlDevRef"=w2012) -> ("MotorControlDevRef"=w2003:T7)  [unwired: 7 in, 2 out]
      }
      n523 = flat-sequence {
        tunnel: [w1984] -> w1937
        tunnel: [w1983] -> w1936
        tunnel: [w1982] -> w1935
        tunnel: [w1981] -> w1934
        tunnel: w1941 -> [w1980]
        tunnel: w1940 -> [w1979]
        tunnel: w1939 -> [w1978]
        tunnel: w1938 -> [w1977]
        frame #0 {
          n524 = while {
            tunnel: [w1994] -> w1981
            tunnel: w1980 -> [w1999]
            tunnel: [w1992] -> w1982
            tunnel: w1979 -> [w1998]
            tunnel: [w1997] -> w1983
            tunnel: w1978 -> [w1997]
            tunnel: [w1990] -> w1984
            tunnel: w1977 -> [w1996]
            i -> [w1988]
            stop <- w1985 stop-if-true
            # "1 Sec."
            # "Stop Motors, Shooter Down."
            n525 = Increment(x=w1988) -> (x+1=w1987:i32)
            n526 = call <vilib>:"WPI_MotorControlSetOutput.vi"("Output"=0.0, "MotorControlDevRef"=w1999) -> ("MotorControlDevRef"=w1994:T7)  [unwired: 7 in, 2 out]
            n527 = Wait (ms)(milliseconds to wait=u32 25) -> ()  [unwired: 1 out]
            n528 = Greater Or Equal?(x=w1987, y=40) -> (x >= y?=w1985:bool)
            n529 = call-poly <vilib>:"WPI_SolenoidSet.vi"("Value"=WPI_SolenoidValue."Reverse", "SolenoidDevRef"=w1996) -> ("SolenoidDevRef"=w1990:T4)  [unwired: 8 in, 1 out]
            n530 = call <vilib>:"WPI_MotorControlSetOutput.vi"("Output"=0.0, "MotorControlDevRef"=w1998) -> ("MotorControlDevRef"=w1992:T7)  [unwired: 7 in, 2 out]
          }
        }
      }
      n531 = while {
        tunnel: [w1976] -> _
        tunnel: w1937 -> [w1976]
        tunnel: [w1972] -> _
        tunnel: w1936 -> [w1975]
        tunnel: [w1974] -> _
        tunnel: w1935 -> [w1974]
        tunnel: [w1973] -> _
        tunnel: w1934 -> [w1973]
        i -> [w1969]
        stop <- w1966 stop-if-true
        # "Total Time: 13 Sec."
        # "1 Sec."
        # "Lift-Kit Down"
        n532 = Increment(x=w1969) -> (x+1=w1968:i32)
        n533 = Wait (ms)(milliseconds to wait=u32 25) -> ()  [unwired: 1 out]
        n534 = Greater Or Equal?(x=w1968, y=40) -> (x >= y?=w1966:bool)
        n535 = call-poly <vilib>:"WPI_SolenoidSet.vi"("Value"=WPI_SolenoidValue."Reverse", "SolenoidDevRef"=w1975) -> ("SolenoidDevRef"=w1972:T4)  [unwired: 8 in, 1 out]
      }
    }
    frame "Demo Code" {
      n536 = call <vilib>:"WPI_MotorControlRefNum Registry Get.vi"("refnum name"="Top Motor") -> ("MotorControlDevRef"=w2072:T7)  [unwired: 9 in, 1 out]
      n537 = call <vilib>:"WPI_MotorControlRefNum Registry Get.vi"("refnum name"="Bottom Motor") -> ("MotorControlDevRef"=w2071:T7)  [unwired: 9 in, 1 out]
      n538 = call <vilib>:"WPI_DigitalInputRefNum Registry Get.vi"("refnum name"="Front Limit Switch") -> ("DigitalInputDevRef"=w2068:T14)  [unwired: 9 in, 1 out]
      n539 = while {
        tunnel: [w2081] -> _
        tunnel: w2072 -> [w2083]
        tunnel: [w2079] -> _
        tunnel: w2071 -> [w2082]
        tunnel: w2068 -> [w2076]
        stop <- w2073 stop-if-true
        n540 = Wait (ms)(milliseconds to wait=u32 25) -> ()  [unwired: 1 out]
        n541 = call <vilib>:"WPI_MotorControlSetOutput.vi"("Output"=0.08, "MotorControlDevRef"=w2083) -> ("MotorControlDevRef"=w2081:T7)  [unwired: 7 in, 2 out]
        n542 = call <vilib>:"WPI_MotorControlSetOutput.vi"("Output"=0.08, "MotorControlDevRef"=w2082) -> ("MotorControlDevRef"=w2079:T7)  [unwired: 7 in, 2 out]
        n543 = call <vilib>:"WPI_DigitalInputGetValue.vi"("DigitalInputDevRef"=w2076) -> ("Value"=w2075:bool)  [unwired: 8 in, 2 out]
        n544 = Equal?(x=w2075, y=TRUE) -> (x = y?=w2073:bool)
      }
    }
    frame "Gyro Testing" {
      n545 = call <vilib>:"WPI_RobotDriveRefNum Registry Get.vi"("refnum name"="Left and Right Motors") -> ("RobotDriveDevRef"=w2086:T6)  [unwired: 9 in, 1 out]
      n546 = while {
        tunnel: w2086 -> [w2112]
        tunnel: [w2106] -> w2085
        stop <- w2107 stop-if-true
        n547 = global read "Robot Global Data.vi" "Gyro angle"() -> (w2109:dbl)
        n548 = call <vilib>:"WPI_RobotDriveTankDrive.vi"("Right axis value"=-0.7, "Left axis value"=0.7, "RobotDriveDevRef"=w2112) -> ("RobotDriveDevRef"=w2106:T6)  [unwired: 6 in, 2 out]
        n549 = Greater Or Equal?(x=w2109, y=90.0) -> (x >= y?=w2107:bool)
        n550 = Wait (ms)(milliseconds to wait=u32 25) -> ()  [unwired: 1 out]
      }
      n551 = while {
        tunnel: w2085 -> [w2104]
        tunnel: [w2096] -> w2084
        i -> [w2100]
        stop <- w2097 stop-if-true
        # "Wait 2 Sec."
        n552 = call <vilib>:"WPI_RobotDriveTankDrive.vi"("Right axis value"=0.0, "Left axis value"=0.0, "RobotDriveDevRef"=w2104) -> ("RobotDriveDevRef"=w2096:T6)  [unwired: 6 in, 2 out]
        n553 = Increment(x=w2100) -> (x+1=w2099:i32)
        n554 = Greater Or Equal?(x=w2099, y=80) -> (x >= y?=w2097:bool)
        n555 = Wait (ms)(milliseconds to wait=u32 25) -> ()  [unwired: 1 out]
      }
      n556 = while {
        tunnel: w2084 -> [w2095]
        tunnel: [w2089] -> _
        stop <- w2090 stop-if-true
        n557 = global read "Robot Global Data.vi" "Gyro angle"() -> (w2092:dbl)
        n558 = call <vilib>:"WPI_RobotDriveTankDrive.vi"("Right axis value"=-0.7, "Left axis value"=0.7, "RobotDriveDevRef"=w2095) -> ("RobotDriveDevRef"=w2089:T6)  [unwired: 6 in, 2 out]
        n559 = Greater Or Equal?(x=w2092, y=-90.0) -> (x >= y?=w2090:bool)
        n560 = Wait (ms)(milliseconds to wait=u32 25) -> ()  [unwired: 1 out]
      }
    }
  }
  n561 = Index Array(array=w2, index=2) -> ()  [unwired: 1 out]
  n562 = call-poly <vilib>:"NT Write Value.vi"("Numeric Array"=w2, "Name"="Joystick 0/Axes") -> ()  [unwired: 9 in, 1 out]
